vi "函数类型1测试.vi"() -> ()   [LabVIEW 2010]
uses:
  全局量/试验配置信息.vi
panel:
  out "starttest":bool
  out "bRece":bool
  out "bSend":bool
  out "D_IN_1":string[][](table) caption="表格"
  in  "加载文件名称":string
  out "配置文件路径":path
  out "配置文件目录":path
  in  "同步_1":i32
  in  "数组_反馈值":dbl[][](array[numeric])
  in  "第几个数据":i32
  in  "第几组数据":i32
  in  "数组_设定值":dbl[][](array[numeric])
  in  "数组_选择":bool[](array[boolean])
  out "light_32":bool
  out "light_31":bool
  out "light_30":bool
  out "light_29":bool
  out "light_28":bool
  out "light_27":bool
  out "light_26":bool
  out "light_25":bool
  out "light_24":bool
  out "light_23":bool
  out "light_22":bool
  out "light_21":bool
  out "light_20":bool
  out "light_19":bool
  out "light_18":bool
  out "light_17":bool
  out "Analog_back":string[][](table) caption="表格"
  in  "A_32":bool
  in  "A_31":bool
  in  "A_30":bool
  in  "A_29":bool
  in  "A_28":bool
  in  "A_27":bool
  in  "A_26":bool
  in  "A_25":bool
  in  "A_24":bool
  in  "A_23":bool
  in  "A_22":bool
  in  "A_21":bool
  in  "A_20":bool
  in  "A_19":bool
  in  "A_18":bool
  in  "A_17":bool
  out "合格？":bool[][](array[boolean])
  out "测试结论":string
  out "light_16":bool
  out "light_15":bool
  out "light_14":bool
  out "light_13":bool
  out "light_12":bool
  out "light_11":bool
  out "light_10":bool
  out "light_9":bool
  out "light_8":bool
  out "light_7":bool
  out "light_6":bool
  out "light_5":bool
  out "light_4":bool
  out "light_3":bool
  out "light_2":bool
  out "light_1":bool
  out "退出？":bool
  in  "btn_反选":bool
  in  "btn_全选":bool
  in  "A_16":bool
  in  "A_15":bool
  in  "A_14":bool
  in  "A_13":bool
  in  "A_12":bool
  in  "A_11":bool
  in  "A_10":bool
  in  "A_9":bool
  in  "A_8":bool
  in  "A_7":bool
  in  "A_6":bool
  in  "A_5":bool
  in  "A_4":bool
  in  "A_3":bool
  in  "A_2":bool
  in  "A_1":bool
  in  "btn_取消":bool
  in  "btn_开始测试":bool
  in  "Analog_IN":string[][](table) caption="表格"
  out "Analog_WC":string[][](table) caption="表格"
  # "模拟量选择及输入值（V）"
  # "模拟量反馈值（V）"
  # "模拟量误差值（%）"
  # "测试结论："
  # "从0开始"
  # "从1开始,第0列没有使用"
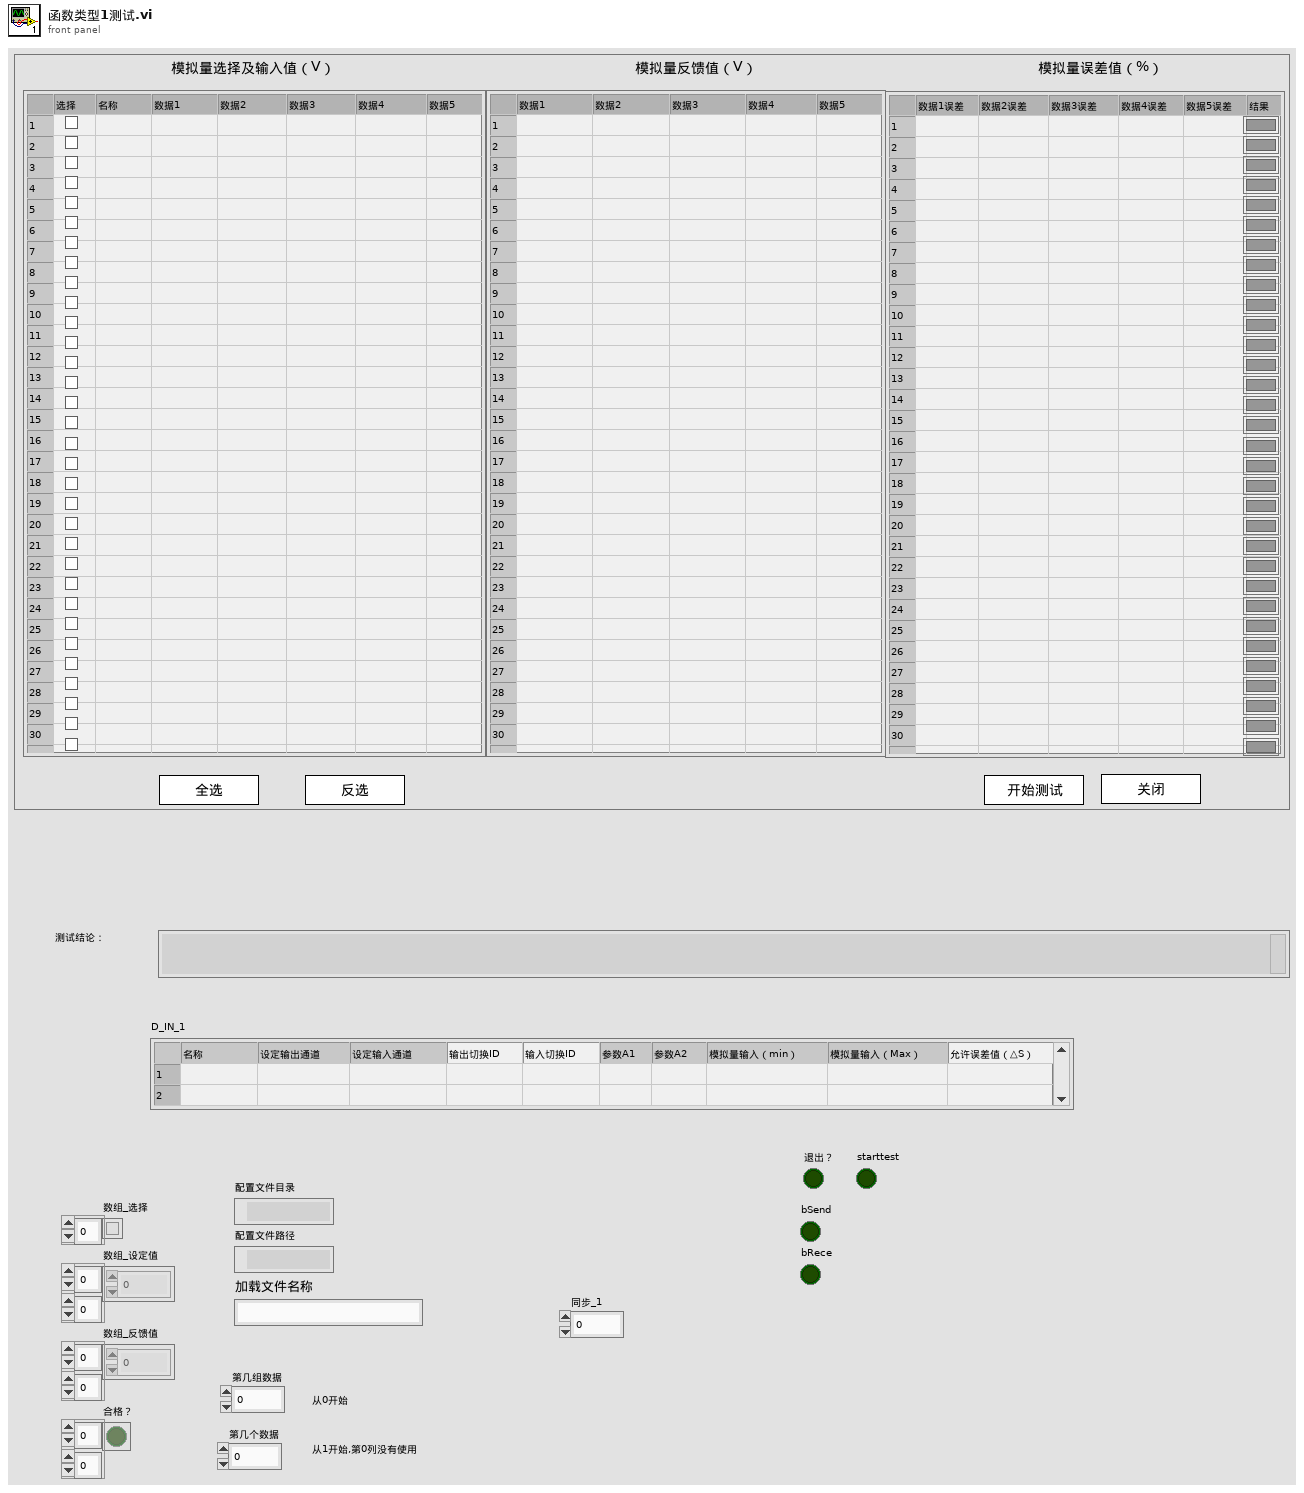
[diagram p1: front panel]
types:
  T1 = enum8{"Enabled", "Disabled", "Disabled and Grayed Out"}
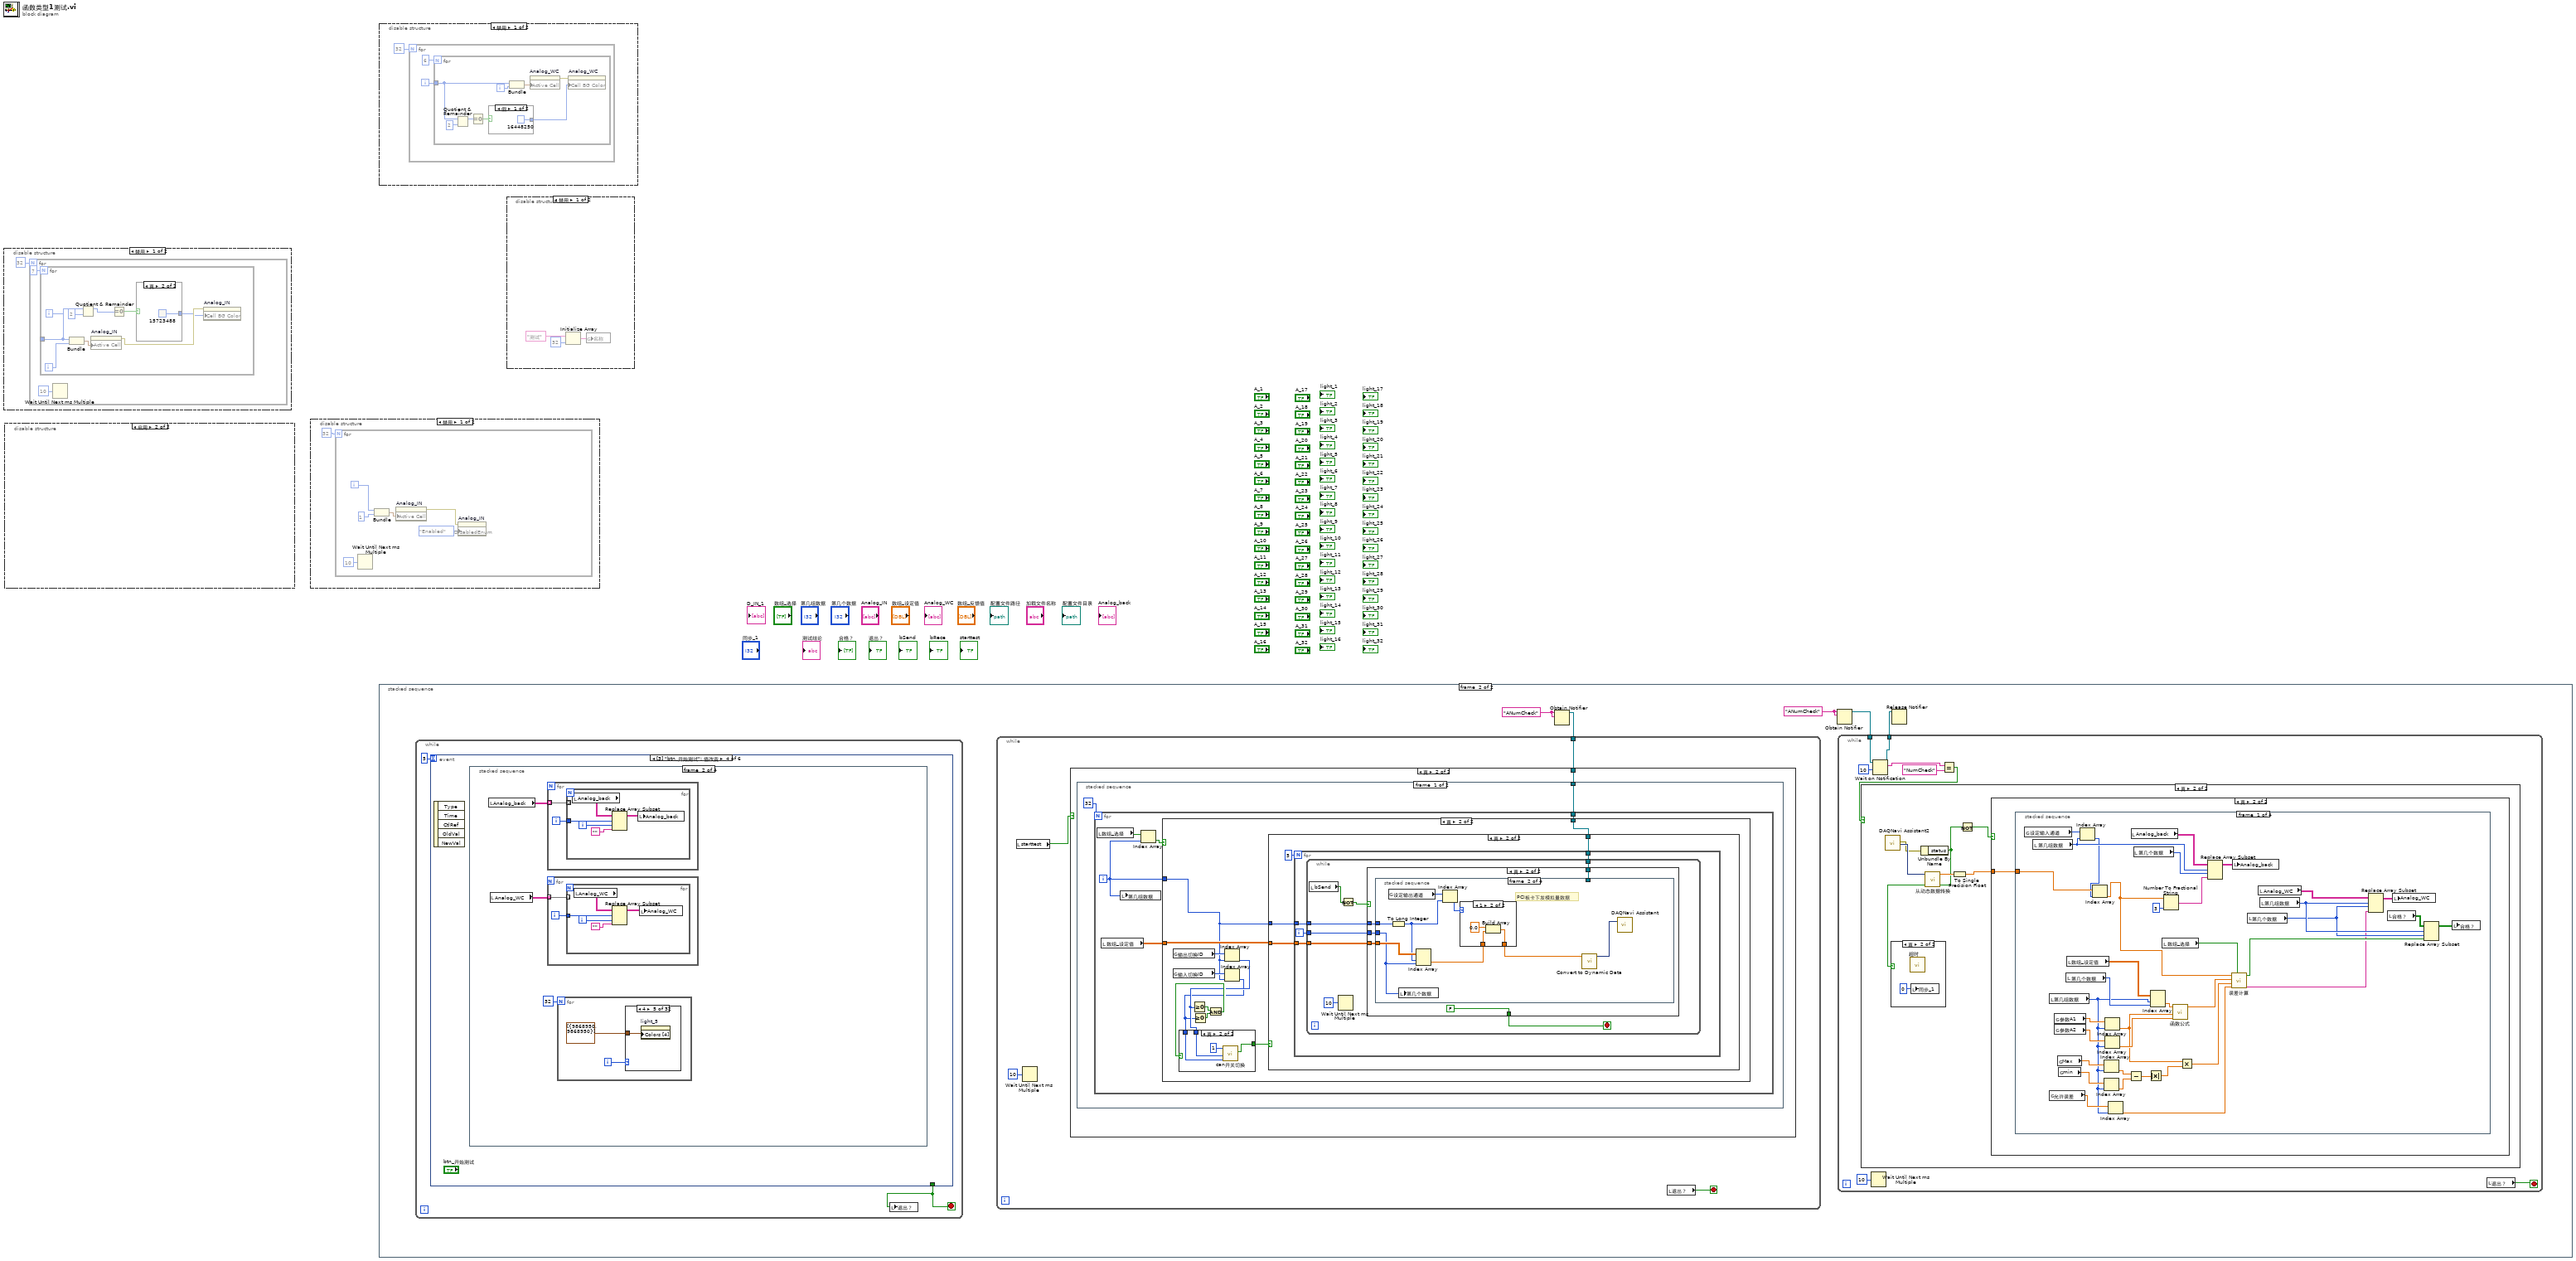
[diagram p0: block diagram]
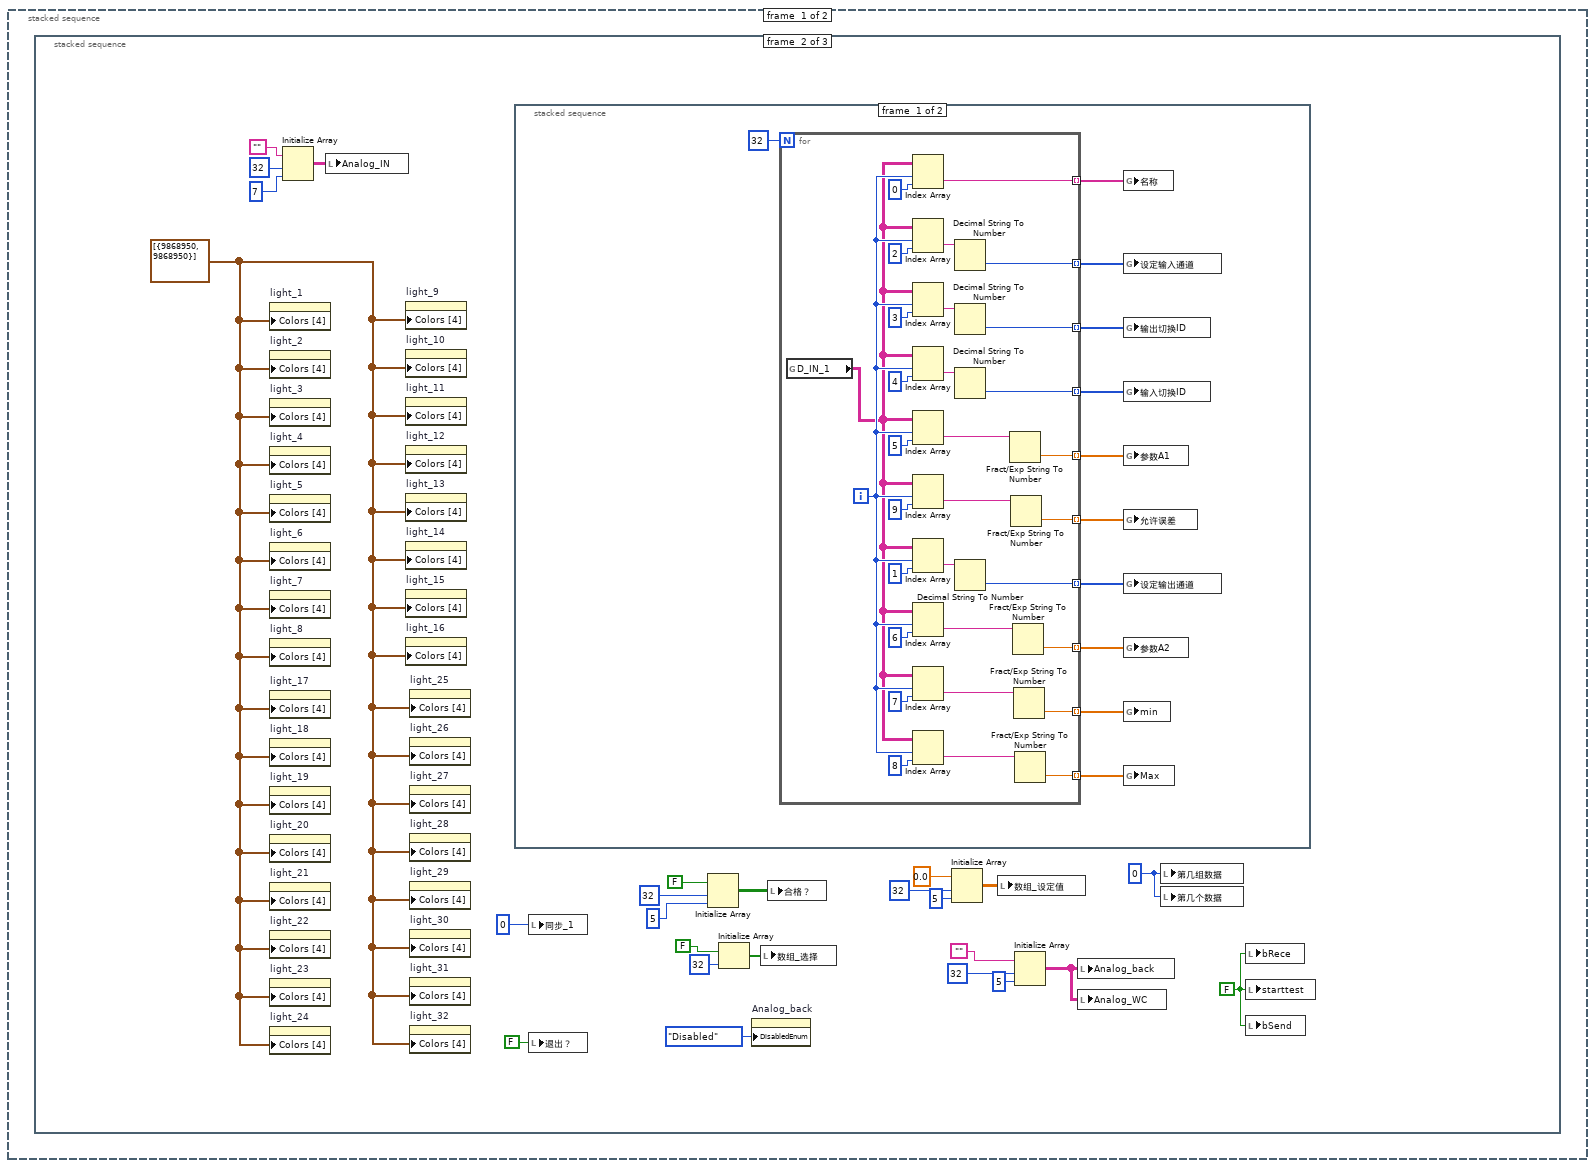
[diagram p2: hidden frame]
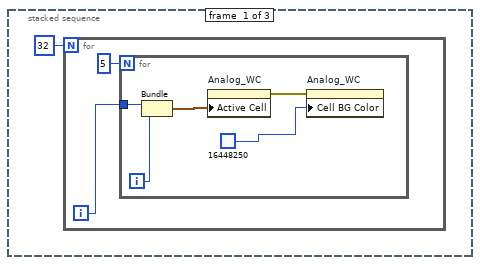
[diagram p3: hidden frame]
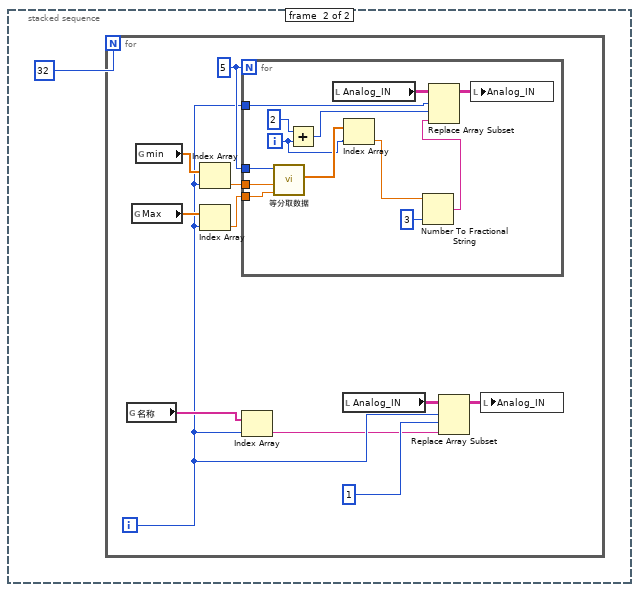
[diagram p4: hidden frame]
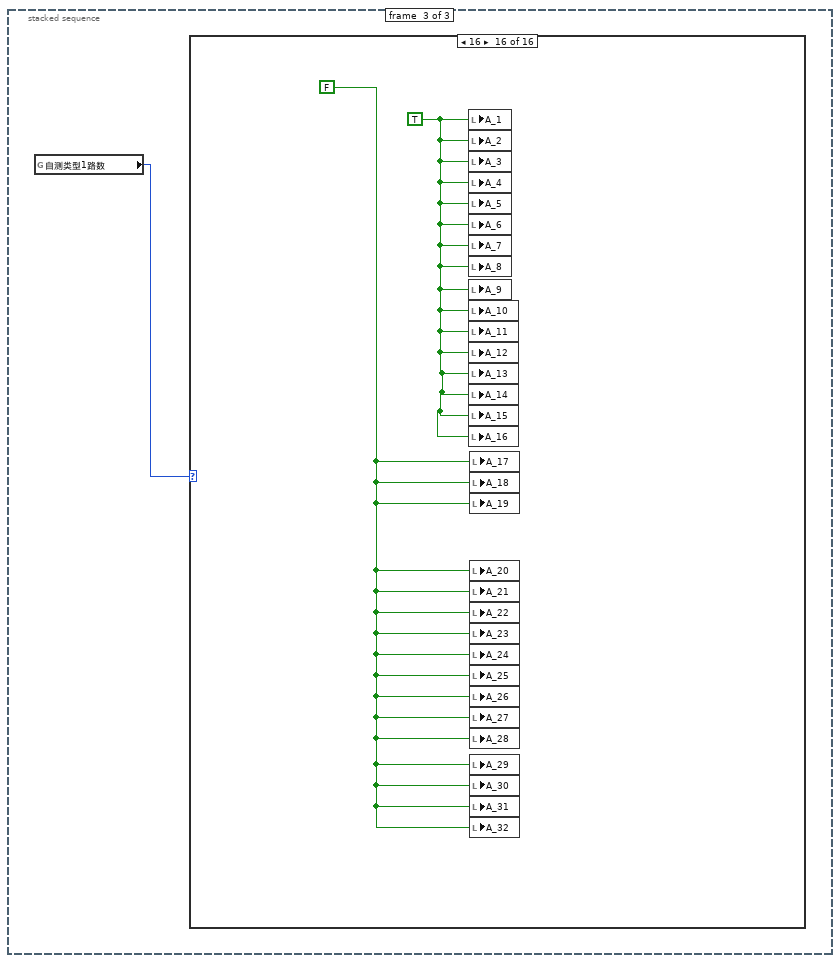
[diagram p5: hidden frame]
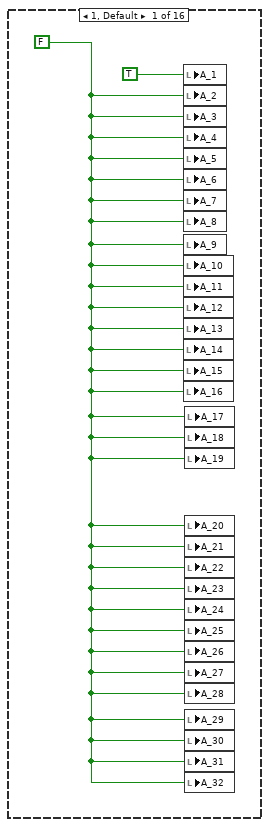
[diagram p6: hidden frame]
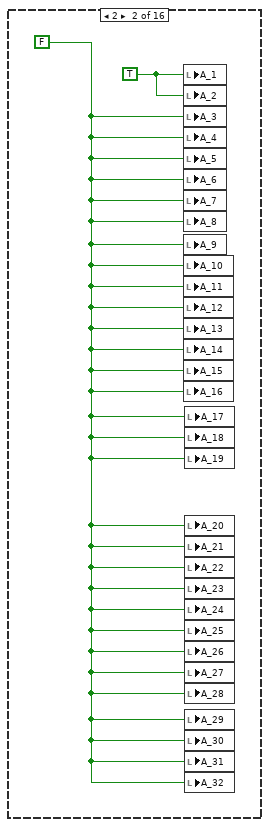
[diagram p7: hidden frame]
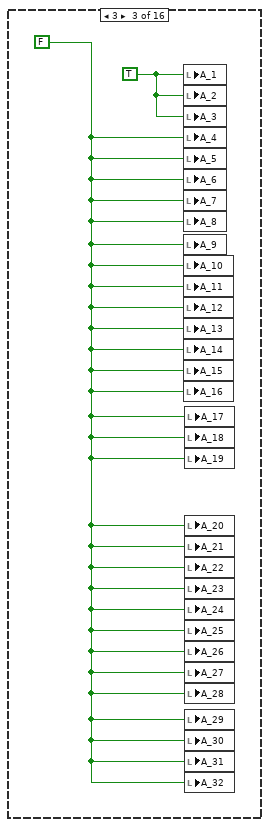
[diagram p8: hidden frame]
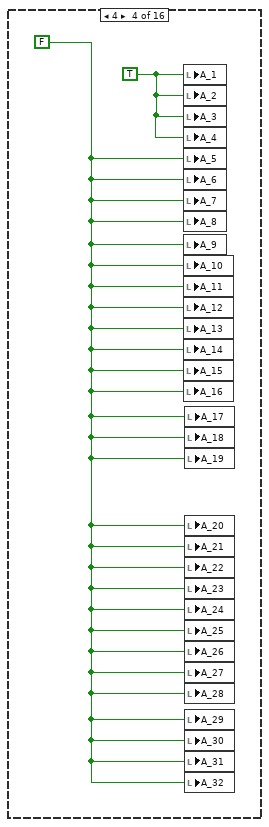
[diagram p9: hidden frame]
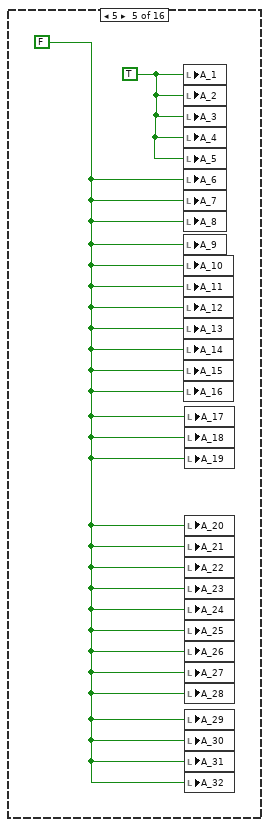
[diagram p10: hidden frame]
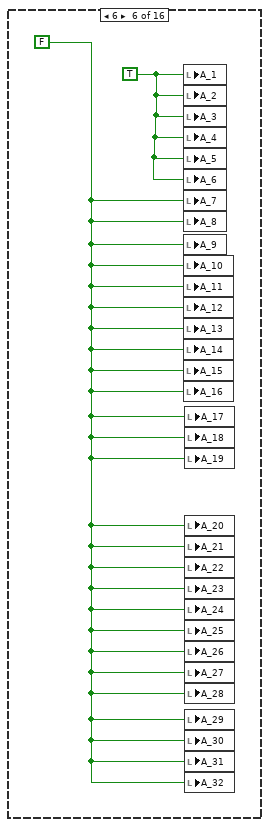
[diagram p11: hidden frame]
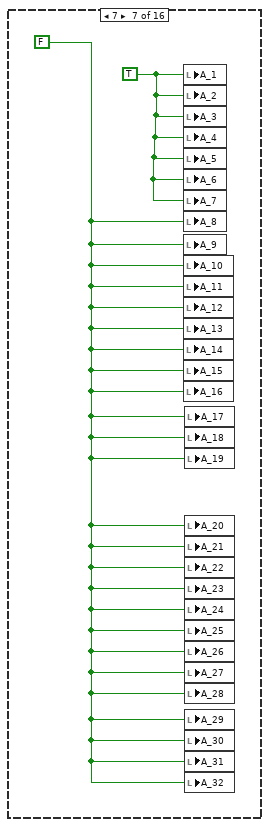
[diagram p12: hidden frame]
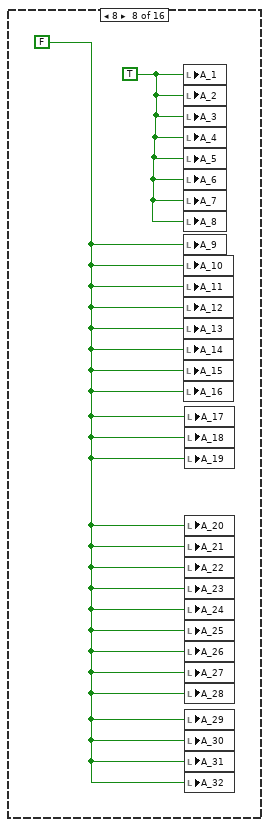
[diagram p13: hidden frame]
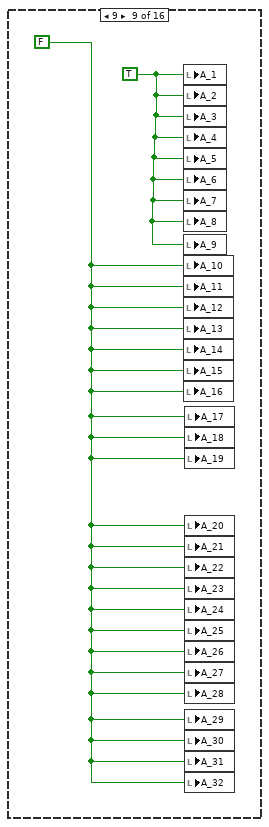
[diagram p14: hidden frame]
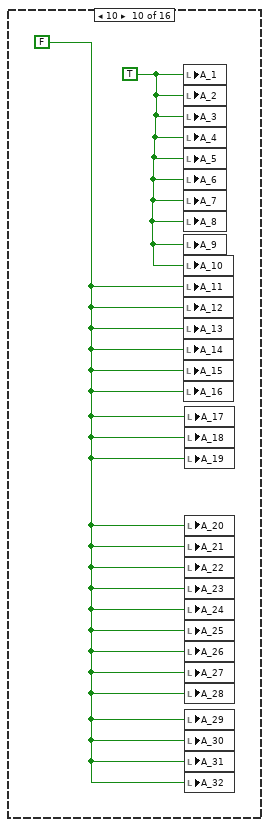
[diagram p15: hidden frame]
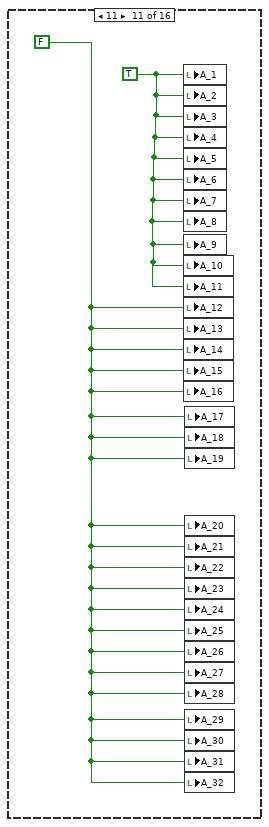
[diagram p16: hidden frame]
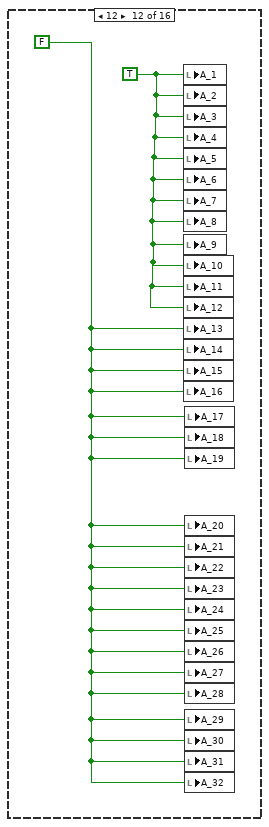
[diagram p17: hidden frame]
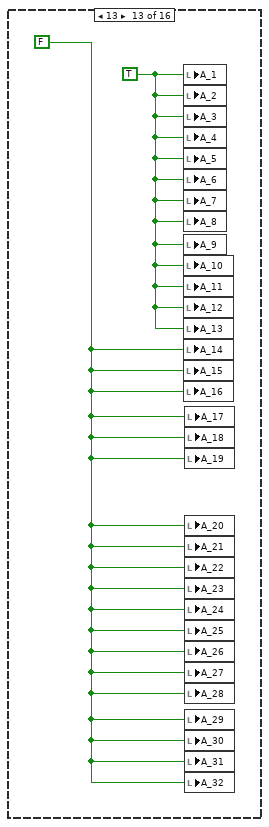
[diagram p18: hidden frame]
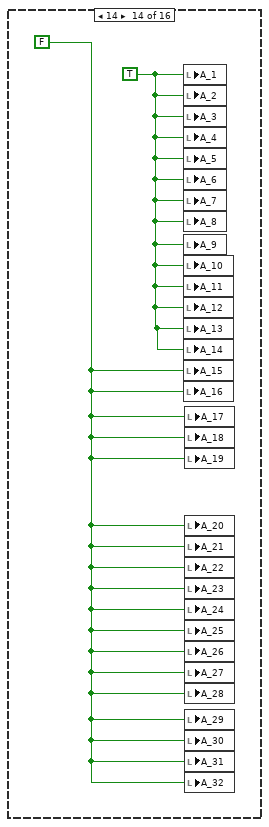
[diagram p19: hidden frame]
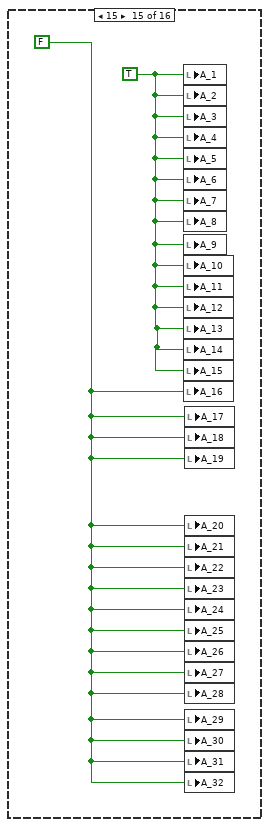
[diagram p20: hidden frame]
diagram:
  n1 = disable-structure shown="禁用" {
    frame Disabled {
      n2 = for {
        N: 32 -> [_]
        i -> [w3]
        n3 = for {
          N: 7 -> [_]
          tunnel: w3 -> [w11]
          i -> [w5]
          n4 = Bundle(w11, w5) -> (w8:cluster{i32, i32})  [unwired: 1 in]
          n5 = Quotient & Remainder(x=w11, y=2) -> (x-y*floor(x/y)=w9:i32)  [unwired: 1 out]
          n6 = property on="Analog_IN" class="Tbl (严格)"("Active Cell"=w8) -> (error out=w7:errorcluster)  [unwired: 2 in, 1 out]
          n7 = Equal To 0?(x=w9) -> (x = 0?=w12:bool)
          n8 = case shown="真" w12 {
            tunnel: [u32 16448250 u32 15723488] -> w6
            frame False {
            }
            frame True {
            }
          }
          n9 = property on="Analog_IN" class="Tbl (严格)"(error in=w7, "Cell BG Color"=w6) -> ()  [unwired: 1 in, 2 out]
        }
        n10 = Wait Until Next ms Multiple(millisecond multiple=u32 10 ("毫秒倍数")) -> ()  [unwired: 1 out]
      }
    }
    frame Enabled {
    }
  }
  n11 = disable-structure shown="启用" {
    frame Disabled {
      n12 = for {
        N: 32 -> [_]
        i -> [w16]
        n13 = for {
          N: 7 -> [_]
          tunnel: w16 -> [w19]
          i -> [w20]
          n14 = Bundle(w19, w20) -> (w23:cluster{i32, i32})  [unwired: 1 in]
          n15 = property on="Analog_IN" class="Tbl (严格)"("Active Cell"=w23) -> (error out=w21:errorcluster)  [unwired: 2 in, 1 out]
          n16 = property on="Analog_IN" class="Tbl (严格)"(error in=w21, "Justify"=enum16{"Left", "Center", "Right"}."Left" ("活动单元格:单元格对齐")) -> ()  [unwired: 1 in, 2 out]
        }
        n17 = Wait Until Next ms Multiple(millisecond multiple=u32 10 ("毫秒倍数")) -> ()  [unwired: 1 out]
      }
    }
    frame Enabled {
    }
  }
  n18 = disable-structure shown="禁用" {
    frame Disabled {
      n19 = for {
        N: 32 -> [_]
        i -> [w29]
        n20 = Wait Until Next ms Multiple(millisecond multiple=u32 10 ("毫秒倍数")) -> ()  [unwired: 1 out]
        n21 = Bundle(w29, 1) -> (w28:cluster{i32, i32})  [unwired: 1 in]
        n22 = property on="Analog_IN" class="Tbl (严格)"("Active Cell"=w28) -> (error out=w25:errorcluster)  [unwired: 2 in, 1 out]
        n23 = property on="Analog_IN" class="Tbl (严格)"(error in=w25, "DisabledEnum"=T1."Enabled" ("禁用")) -> ()  [unwired: 1 in, 2 out]
      }
    }
    frame Enabled {
    }
  }
  n24 = stacked-sequence {
    frame #0 {
      n25 = stacked-sequence {
        frame #0 {
          n26 = for {
            N: 32 -> [_]
            i -> [w32]
            n27 = for {
              N: 5 -> [_]
              tunnel: w32 -> [w35]
              i -> [w34]
              n28 = Bundle(w35, w34) -> (w36:cluster{i32, i32})  [unwired: 1 in]
              n29 = property on="Analog_WC" class="Tbl (严格)"("Active Cell"=w36) -> (error out=w38:errorcluster)  [unwired: 2 in, 1 out]
              n30 = property on="Analog_WC" class="Tbl (严格)"(error in=w38, "Cell BG Color"=u32 16448250) -> ()  [unwired: 1 in, 2 out]
            }
          }
        }
        frame #1 {
          w63 = FALSE
          w58 = 0 ("第几组数据")
          w43 = cluster{u32, u32}[] [{9868950, 9868950}]
          n31 = property on="light_1" class="Bool (严格)"("Colors [4]"=w43) -> ()  [unwired: 2 in, 2 out]
          n32 = property on="light_2" class="Bool (严格)"("Colors [4]"=w43) -> ()  [unwired: 2 in, 2 out]
          n33 = property on="light_3" class="Bool (严格)"("Colors [4]"=w43) -> ()  [unwired: 2 in, 2 out]
          n34 = property on="light_4" class="Bool (严格)"("Colors [4]"=w43) -> ()  [unwired: 2 in, 2 out]
          n35 = property on="light_5" class="Bool (严格)"("Colors [4]"=w43) -> ()  [unwired: 2 in, 2 out]
          n36 = property on="light_6" class="Bool (严格)"("Colors [4]"=w43) -> ()  [unwired: 2 in, 2 out]
          n37 = property on="light_7" class="Bool (严格)"("Colors [4]"=w43) -> ()  [unwired: 2 in, 2 out]
          n38 = property on="light_8" class="Bool (严格)"("Colors [4]"=w43) -> ()  [unwired: 2 in, 2 out]
          n39 = property on="light_17" class="Bool (严格)"("Colors [4]"=w43) -> ()  [unwired: 2 in, 2 out]
          n40 = property on="light_18" class="Bool (严格)"("Colors [4]"=w43) -> ()  [unwired: 2 in, 2 out]
          n41 = property on="light_19" class="Bool (严格)"("Colors [4]"=w43) -> ()  [unwired: 2 in, 2 out]
          n42 = property on="light_20" class="Bool (严格)"("Colors [4]"=w43) -> ()  [unwired: 2 in, 2 out]
          n43 = property on="light_21" class="Bool (严格)"("Colors [4]"=w43) -> ()  [unwired: 2 in, 2 out]
          n44 = property on="light_22" class="Bool (严格)"("Colors [4]"=w43) -> ()  [unwired: 2 in, 2 out]
          n45 = property on="light_23" class="Bool (严格)"("Colors [4]"=w43) -> ()  [unwired: 2 in, 2 out]
          n46 = property on="light_24" class="Bool (严格)"("Colors [4]"=w43) -> ()  [unwired: 2 in, 2 out]
          n47 = Initialize Array("", 32 ("维数大小"), 7 ("维数大小")) -> (w59:string[][])
          n48 = local write "Analog_IN"(w59) -> ()
          n49 = property on="light_9" class="Bool (严格)"("Colors [4]"=w43) -> ()  [unwired: 2 in, 2 out]
          n50 = property on="light_10" class="Bool (严格)"("Colors [4]"=w43) -> ()  [unwired: 2 in, 2 out]
          n51 = property on="light_11" class="Bool (严格)"("Colors [4]"=w43) -> ()  [unwired: 2 in, 2 out]
          n52 = property on="light_12" class="Bool (严格)"("Colors [4]"=w43) -> ()  [unwired: 2 in, 2 out]
          n53 = property on="light_13" class="Bool (严格)"("Colors [4]"=w43) -> ()  [unwired: 2 in, 2 out]
          n54 = property on="light_14" class="Bool (严格)"("Colors [4]"=w43) -> ()  [unwired: 2 in, 2 out]
          n55 = property on="light_15" class="Bool (严格)"("Colors [4]"=w43) -> ()  [unwired: 2 in, 2 out]
          n56 = property on="light_16" class="Bool (严格)"("Colors [4]"=w43) -> ()  [unwired: 2 in, 2 out]
          n57 = property on="light_25" class="Bool (严格)"("Colors [4]"=w43) -> ()  [unwired: 2 in, 2 out]
          n58 = property on="light_26" class="Bool (严格)"("Colors [4]"=w43) -> ()  [unwired: 2 in, 2 out]
          n59 = property on="light_27" class="Bool (严格)"("Colors [4]"=w43) -> ()  [unwired: 2 in, 2 out]
          n60 = property on="light_28" class="Bool (严格)"("Colors [4]"=w43) -> ()  [unwired: 2 in, 2 out]
          n61 = property on="light_29" class="Bool (严格)"("Colors [4]"=w43) -> ()  [unwired: 2 in, 2 out]
          n62 = property on="light_30" class="Bool (严格)"("Colors [4]"=w43) -> ()  [unwired: 2 in, 2 out]
          n63 = property on="light_31" class="Bool (严格)"("Colors [4]"=w43) -> ()  [unwired: 2 in, 2 out]
          n64 = property on="light_32" class="Bool (严格)"("Colors [4]"=w43) -> ()  [unwired: 2 in, 2 out]
          n65 = stacked-sequence {
            frame #0 {
              n66 = for {
                N: 32 ("维数大小") -> [_]
                tunnel: [w104] -> w68 mode=indexing
                tunnel: [w100] -> w67 mode=indexing
                tunnel: [w98] -> w66 mode=indexing
                tunnel: [w95] -> w65 mode=indexing
                tunnel: [w92] -> w64 mode=indexing
                tunnel: [w89] -> w70 mode=indexing
                tunnel: [w86] -> w71 mode=indexing
                tunnel: [w83] -> w72 mode=indexing
                tunnel: [w80] -> w73 mode=indexing
                tunnel: [w76] -> w74 mode=indexing
                i -> [w78]
                n67 = global read "试验配置信息.vi" "D_IN_1"() -> (w75:string[][])
                n68 = Index Array(array=w75, index (row)=w78, index (col)=0 ("禁用的索引 (列)")) -> (element=w104:string)
                n69 = Index Array(array=w75, index (row)=w78, index (col)=2 ("禁用的索引 (列)")) -> (element=w94:string)
                n70 = Index Array(array=w75, index (row)=w78, index (col)=3 ("禁用的索引 (列)")) -> (element=w90:string)
                n71 = Index Array(array=w75, index (row)=w78, index (col)=4 ("禁用的索引 (列)")) -> (element=w88:string)
                n72 = Index Array(array=w75, index (row)=w78, index (col)=5 ("禁用的索引 (列)")) -> (element=w85:string)
                n73 = Index Array(array=w75, index (row)=w78, index (col)=9 ("禁用的索引 (列)")) -> (element=w77:string)
                n74 = Index Array(array=w75, index (row)=w78, index (col)=1 ("禁用的索引 (列)")) -> (element=w97:string)
                n75 = Index Array(array=w75, index (row)=w78, index (col)=6 ("禁用的索引 (列)")) -> (element=w81:string)
                n76 = Index Array(array=w75, index (row)=w78, index (col)=7 ("禁用的索引 (列)")) -> (element=w101:string)
                n77 = Index Array(array=w75, index (row)=w78, index (col)=8 ("禁用的索引 (列)")) -> (element=w99:string)
                n78 = Decimal String To Number(string=w94) -> (number=w92:i32)  [unwired: 2 in, 1 out]
                n79 = Decimal String To Number(string=w90) -> (number=w89:i32)  [unwired: 2 in, 1 out]
                n80 = Decimal String To Number(string=w88) -> (number=w86:i32)  [unwired: 2 in, 1 out]
                n81 = Decimal String To Number(string=w97) -> (number=w95:i32)  [unwired: 2 in, 1 out]
                n82 = Fract/Exp String To Number(string=w85) -> (number=w83:dbl)  [unwired: 3 in, 1 out]
                n83 = Fract/Exp String To Number(string=w77) -> (number=w76:dbl)  [unwired: 3 in, 1 out]
                n84 = Fract/Exp String To Number(string=w81) -> (number=w80:dbl)  [unwired: 3 in, 1 out]
                n85 = Fract/Exp String To Number(string=w101) -> (number=w100:dbl)  [unwired: 3 in, 1 out]
                n86 = Fract/Exp String To Number(string=w99) -> (number=w98:dbl)  [unwired: 3 in, 1 out]
              }
              n87 = global write "试验配置信息.vi" "名称"(w68) -> ()
              n88 = global write "试验配置信息.vi" "设定输入通道"(w64) -> ()
              n89 = global write "试验配置信息.vi" "输出切换ID"(w70) -> ()
              n90 = global write "试验配置信息.vi" "输入切换ID"(w71) -> ()
              n91 = global write "试验配置信息.vi" "参数A1"(w72) -> ()
              n92 = global write "试验配置信息.vi" "允许误差"(w74) -> ()
              n93 = global write "试验配置信息.vi" "设定输出通道"(w65) -> ()
              n94 = global write "试验配置信息.vi" "参数A2"(w73) -> ()
              n95 = global write "试验配置信息.vi" "min"(w67) -> ()
              n96 = global write "试验配置信息.vi" "Max"(w66) -> ()
            }
            frame #1 {
              n97 = for {
                N: 32 -> [_]
                i -> [w109]
                w113 = 5 ("num")
                n98 = global read "试验配置信息.vi" "名称"() -> (w112:string[])
                n99 = global read "试验配置信息.vi" "Max"() -> (w116:dbl[])
                n100 = global read "试验配置信息.vi" "min"() -> (w117:dbl[])
                n101 = Index Array(array=w117, index=w109) -> (element=w115:dbl)
                n102 = Index Array(array=w116, index=w109) -> (element=w114:dbl)
                n103 = for {
                  N: w113 -> [_]
                  tunnel: w109 -> [w128]
                  tunnel: w115 -> [w125]
                  tunnel: w114 -> [w124]
                  tunnel: w113 -> [w123]
                  i -> [w121]
                  n104 = call "等分取数据.vi"("Max"=w124, "MIN"=w125, "num"=w123) -> ("数据点"=w122:dbl[])  [unwired: 5 in]
                  n105 = Add(x=2, y=w121) -> (x+y=w126:i32)
                  n106 = local read "Analog_IN"() -> (w130:string[][])
                  n107 = Index Array(array=w122, index=w121) -> (element=w119:dbl)
                  n108 = Number To Fractional String(number=w119, precision (6)=i16 3 ("精度(6)")) -> (F-format string=w120:string)  [unwired: 2 in]
                  n109 = Replace Array Subset(array=w130, new element=w120, index (row)=w128, index (col)=w126) -> (w129:string[][])
                  n110 = local write "Analog_IN"(w129) -> ()
                }
                n111 = Index Array(array=w112, index=w109) -> (element=w107:string)
                n112 = local read "Analog_IN"() -> (w110:string[][])
                n113 = Replace Array Subset(array=w110, new element=w107, index (row)=w109, index (col)=1) -> (w111:string[][])
                n114 = local write "Analog_IN"(w111) -> ()
              }
            }
          }
          n115 = local write "同步_1"(0 ("同步_2")) -> ()
          n116 = local write "退出？"(FALSE ("退出？")) -> ()
          n117 = Initialize Array(FALSE, 32 ("维数大小"), 5 ("维数大小")) -> (w42:bool[][])
          n118 = Initialize Array(FALSE, 32 ("维数大小")) -> (w54:bool[])
          n119 = property on="Analog_back" class="Tbl (严格)"("DisabledEnum"=T1."Disabled" ("禁用")) -> ()  [unwired: 2 in, 2 out]
          n120 = local write "数组_选择"(w54) -> ()
          n121 = local write "合格？"(w42) -> ()
          n122 = Initialize Array(0.0, 32 ("维数大小"), 5 ("维数大小")) -> (w51:dbl[][])
          n123 = local write "数组_设定值"(w51) -> ()
          n124 = Initialize Array("", 32 ("维数大小"), 5 ("维数大小")) -> (w47:string[][])
          n125 = local write "Analog_back"(w47) -> ()
          n126 = local write "Analog_WC"(w47) -> ()
          n127 = local write "第几组数据"(w58) -> ()
          n128 = local write "第几个数据"(w58) -> ()
          n129 = local write "bRece"(w63) -> ()
          n130 = local write "starttest"(w63) -> ()
          n131 = local write "bSend"(w63) -> ()
        }
        frame #2 {
          n132 = global read "试验配置信息.vi" "自测类型1路数"() -> (w131:i32)
          n133 = case shown="16" w131 {
            frame 1, Default {
              w133 = FALSE ("单选_AD_1")
              n134 = local write "A_1"(TRUE) -> ()
              n135 = local write "A_2"(w133) -> ()
              n136 = local write "A_3"(w133) -> ()
              n137 = local write "A_4"(w133) -> ()
              n138 = local write "A_5"(w133) -> ()
              n139 = local write "A_6"(w133) -> ()
              n140 = local write "A_7"(w133) -> ()
              n141 = local write "A_8"(w133) -> ()
              n142 = local write "A_9"(w133) -> ()
              n143 = local write "A_10"(w133) -> ()
              n144 = local write "A_11"(w133) -> ()
              n145 = local write "A_12"(w133) -> ()
              n146 = local write "A_13"(w133) -> ()
              n147 = local write "A_14"(w133) -> ()
              n148 = local write "A_15"(w133) -> ()
              n149 = local write "A_16"(w133) -> ()
              n150 = local write "A_17"(w133) -> ()
              n151 = local write "A_18"(w133) -> ()
              n152 = local write "A_19"(w133) -> ()
              n153 = local write "A_20"(w133) -> ()
              n154 = local write "A_21"(w133) -> ()
              n155 = local write "A_22"(w133) -> ()
              n156 = local write "A_23"(w133) -> ()
              n157 = local write "A_24"(w133) -> ()
              n158 = local write "A_25"(w133) -> ()
              n159 = local write "A_26"(w133) -> ()
              n160 = local write "A_27"(w133) -> ()
              n161 = local write "A_28"(w133) -> ()
              n162 = local write "A_29"(w133) -> ()
              n163 = local write "A_30"(w133) -> ()
              n164 = local write "A_31"(w133) -> ()
              n165 = local write "A_32"(w133) -> ()
            }
            frame 2 {
              w134 = TRUE
              w135 = FALSE ("单选_AD_1")
              n166 = local write "A_1"(w134) -> ()
              n167 = local write "A_2"(w134) -> ()
              n168 = local write "A_3"(w135) -> ()
              n169 = local write "A_4"(w135) -> ()
              n170 = local write "A_5"(w135) -> ()
              n171 = local write "A_6"(w135) -> ()
              n172 = local write "A_7"(w135) -> ()
              n173 = local write "A_8"(w135) -> ()
              n174 = local write "A_9"(w135) -> ()
              n175 = local write "A_10"(w135) -> ()
              n176 = local write "A_11"(w135) -> ()
              n177 = local write "A_12"(w135) -> ()
              n178 = local write "A_13"(w135) -> ()
              n179 = local write "A_14"(w135) -> ()
              n180 = local write "A_15"(w135) -> ()
              n181 = local write "A_16"(w135) -> ()
              n182 = local write "A_17"(w135) -> ()
              n183 = local write "A_18"(w135) -> ()
              n184 = local write "A_19"(w135) -> ()
              n185 = local write "A_20"(w135) -> ()
              n186 = local write "A_21"(w135) -> ()
              n187 = local write "A_22"(w135) -> ()
              n188 = local write "A_23"(w135) -> ()
              n189 = local write "A_24"(w135) -> ()
              n190 = local write "A_25"(w135) -> ()
              n191 = local write "A_26"(w135) -> ()
              n192 = local write "A_27"(w135) -> ()
              n193 = local write "A_28"(w135) -> ()
              n194 = local write "A_29"(w135) -> ()
              n195 = local write "A_30"(w135) -> ()
              n196 = local write "A_31"(w135) -> ()
              n197 = local write "A_32"(w135) -> ()
            }
            frame 3 {
              w136 = TRUE
              w137 = FALSE ("单选_AD_1")
              n198 = local write "A_1"(w136) -> ()
              n199 = local write "A_2"(w136) -> ()
              n200 = local write "A_3"(w136) -> ()
              n201 = local write "A_4"(w137) -> ()
              n202 = local write "A_5"(w137) -> ()
              n203 = local write "A_6"(w137) -> ()
              n204 = local write "A_7"(w137) -> ()
              n205 = local write "A_8"(w137) -> ()
              n206 = local write "A_9"(w137) -> ()
              n207 = local write "A_10"(w137) -> ()
              n208 = local write "A_11"(w137) -> ()
              n209 = local write "A_12"(w137) -> ()
              n210 = local write "A_13"(w137) -> ()
              n211 = local write "A_14"(w137) -> ()
              n212 = local write "A_15"(w137) -> ()
              n213 = local write "A_16"(w137) -> ()
              n214 = local write "A_17"(w137) -> ()
              n215 = local write "A_18"(w137) -> ()
              n216 = local write "A_19"(w137) -> ()
              n217 = local write "A_20"(w137) -> ()
              n218 = local write "A_21"(w137) -> ()
              n219 = local write "A_22"(w137) -> ()
              n220 = local write "A_23"(w137) -> ()
              n221 = local write "A_24"(w137) -> ()
              n222 = local write "A_25"(w137) -> ()
              n223 = local write "A_26"(w137) -> ()
              n224 = local write "A_27"(w137) -> ()
              n225 = local write "A_28"(w137) -> ()
              n226 = local write "A_29"(w137) -> ()
              n227 = local write "A_30"(w137) -> ()
              n228 = local write "A_31"(w137) -> ()
              n229 = local write "A_32"(w137) -> ()
            }
            frame 4 {
              w138 = TRUE
              w139 = FALSE ("单选_AD_1")
              n230 = local write "A_1"(w138) -> ()
              n231 = local write "A_2"(w138) -> ()
              n232 = local write "A_3"(w138) -> ()
              n233 = local write "A_4"(w138) -> ()
              n234 = local write "A_5"(w139) -> ()
              n235 = local write "A_6"(w139) -> ()
              n236 = local write "A_7"(w139) -> ()
              n237 = local write "A_8"(w139) -> ()
              n238 = local write "A_9"(w139) -> ()
              n239 = local write "A_10"(w139) -> ()
              n240 = local write "A_11"(w139) -> ()
              n241 = local write "A_12"(w139) -> ()
              n242 = local write "A_13"(w139) -> ()
              n243 = local write "A_14"(w139) -> ()
              n244 = local write "A_15"(w139) -> ()
              n245 = local write "A_16"(w139) -> ()
              n246 = local write "A_17"(w139) -> ()
              n247 = local write "A_18"(w139) -> ()
              n248 = local write "A_19"(w139) -> ()
              n249 = local write "A_20"(w139) -> ()
              n250 = local write "A_21"(w139) -> ()
              n251 = local write "A_22"(w139) -> ()
              n252 = local write "A_23"(w139) -> ()
              n253 = local write "A_24"(w139) -> ()
              n254 = local write "A_25"(w139) -> ()
              n255 = local write "A_26"(w139) -> ()
              n256 = local write "A_27"(w139) -> ()
              n257 = local write "A_28"(w139) -> ()
              n258 = local write "A_29"(w139) -> ()
              n259 = local write "A_30"(w139) -> ()
              n260 = local write "A_31"(w139) -> ()
              n261 = local write "A_32"(w139) -> ()
            }
            frame 5 {
              w140 = TRUE
              w141 = FALSE ("单选_AD_1")
              n262 = local write "A_1"(w140) -> ()
              n263 = local write "A_2"(w140) -> ()
              n264 = local write "A_3"(w140) -> ()
              n265 = local write "A_4"(w140) -> ()
              n266 = local write "A_5"(w140) -> ()
              n267 = local write "A_6"(w141) -> ()
              n268 = local write "A_7"(w141) -> ()
              n269 = local write "A_8"(w141) -> ()
              n270 = local write "A_9"(w141) -> ()
              n271 = local write "A_10"(w141) -> ()
              n272 = local write "A_11"(w141) -> ()
              n273 = local write "A_12"(w141) -> ()
              n274 = local write "A_13"(w141) -> ()
              n275 = local write "A_14"(w141) -> ()
              n276 = local write "A_15"(w141) -> ()
              n277 = local write "A_16"(w141) -> ()
              n278 = local write "A_17"(w141) -> ()
              n279 = local write "A_18"(w141) -> ()
              n280 = local write "A_19"(w141) -> ()
              n281 = local write "A_20"(w141) -> ()
              n282 = local write "A_21"(w141) -> ()
              n283 = local write "A_22"(w141) -> ()
              n284 = local write "A_23"(w141) -> ()
              n285 = local write "A_24"(w141) -> ()
              n286 = local write "A_25"(w141) -> ()
              n287 = local write "A_26"(w141) -> ()
              n288 = local write "A_27"(w141) -> ()
              n289 = local write "A_28"(w141) -> ()
              n290 = local write "A_29"(w141) -> ()
              n291 = local write "A_30"(w141) -> ()
              n292 = local write "A_31"(w141) -> ()
              n293 = local write "A_32"(w141) -> ()
            }
            frame 6 {
              w142 = TRUE
              w143 = FALSE ("单选_AD_1")
              n294 = local write "A_1"(w142) -> ()
              n295 = local write "A_2"(w142) -> ()
              n296 = local write "A_3"(w142) -> ()
              n297 = local write "A_4"(w142) -> ()
              n298 = local write "A_5"(w142) -> ()
              n299 = local write "A_6"(w142) -> ()
              n300 = local write "A_7"(w143) -> ()
              n301 = local write "A_8"(w143) -> ()
              n302 = local write "A_9"(w143) -> ()
              n303 = local write "A_10"(w143) -> ()
              n304 = local write "A_11"(w143) -> ()
              n305 = local write "A_12"(w143) -> ()
              n306 = local write "A_13"(w143) -> ()
              n307 = local write "A_14"(w143) -> ()
              n308 = local write "A_15"(w143) -> ()
              n309 = local write "A_16"(w143) -> ()
              n310 = local write "A_17"(w143) -> ()
              n311 = local write "A_18"(w143) -> ()
              n312 = local write "A_19"(w143) -> ()
              n313 = local write "A_20"(w143) -> ()
              n314 = local write "A_21"(w143) -> ()
              n315 = local write "A_22"(w143) -> ()
              n316 = local write "A_23"(w143) -> ()
              n317 = local write "A_24"(w143) -> ()
              n318 = local write "A_25"(w143) -> ()
              n319 = local write "A_26"(w143) -> ()
              n320 = local write "A_27"(w143) -> ()
              n321 = local write "A_28"(w143) -> ()
              n322 = local write "A_29"(w143) -> ()
              n323 = local write "A_30"(w143) -> ()
              n324 = local write "A_31"(w143) -> ()
              n325 = local write "A_32"(w143) -> ()
            }
            frame 7 {
              w144 = TRUE
              w145 = FALSE ("单选_AD_1")
              n326 = local write "A_1"(w144) -> ()
              n327 = local write "A_2"(w144) -> ()
              n328 = local write "A_3"(w144) -> ()
              n329 = local write "A_4"(w144) -> ()
              n330 = local write "A_5"(w144) -> ()
              n331 = local write "A_6"(w144) -> ()
              n332 = local write "A_7"(w144) -> ()
              n333 = local write "A_8"(w145) -> ()
              n334 = local write "A_9"(w145) -> ()
              n335 = local write "A_10"(w145) -> ()
              n336 = local write "A_11"(w145) -> ()
              n337 = local write "A_12"(w145) -> ()
              n338 = local write "A_13"(w145) -> ()
              n339 = local write "A_14"(w145) -> ()
              n340 = local write "A_15"(w145) -> ()
              n341 = local write "A_16"(w145) -> ()
              n342 = local write "A_17"(w145) -> ()
              n343 = local write "A_18"(w145) -> ()
              n344 = local write "A_19"(w145) -> ()
              n345 = local write "A_20"(w145) -> ()
              n346 = local write "A_21"(w145) -> ()
              n347 = local write "A_22"(w145) -> ()
              n348 = local write "A_23"(w145) -> ()
              n349 = local write "A_24"(w145) -> ()
              n350 = local write "A_25"(w145) -> ()
              n351 = local write "A_26"(w145) -> ()
              n352 = local write "A_27"(w145) -> ()
              n353 = local write "A_28"(w145) -> ()
              n354 = local write "A_29"(w145) -> ()
              n355 = local write "A_30"(w145) -> ()
              n356 = local write "A_31"(w145) -> ()
              n357 = local write "A_32"(w145) -> ()
            }
            frame 8 {
              w146 = TRUE
              w147 = FALSE ("单选_AD_1")
              n358 = local write "A_1"(w146) -> ()
              n359 = local write "A_2"(w146) -> ()
              n360 = local write "A_3"(w146) -> ()
              n361 = local write "A_4"(w146) -> ()
              n362 = local write "A_5"(w146) -> ()
              n363 = local write "A_6"(w146) -> ()
              n364 = local write "A_7"(w146) -> ()
              n365 = local write "A_8"(w146) -> ()
              n366 = local write "A_9"(w147) -> ()
              n367 = local write "A_10"(w147) -> ()
              n368 = local write "A_11"(w147) -> ()
              n369 = local write "A_12"(w147) -> ()
              n370 = local write "A_13"(w147) -> ()
              n371 = local write "A_14"(w147) -> ()
              n372 = local write "A_15"(w147) -> ()
              n373 = local write "A_16"(w147) -> ()
              n374 = local write "A_17"(w147) -> ()
              n375 = local write "A_18"(w147) -> ()
              n376 = local write "A_19"(w147) -> ()
              n377 = local write "A_20"(w147) -> ()
              n378 = local write "A_21"(w147) -> ()
              n379 = local write "A_22"(w147) -> ()
              n380 = local write "A_23"(w147) -> ()
              n381 = local write "A_24"(w147) -> ()
              n382 = local write "A_25"(w147) -> ()
              n383 = local write "A_26"(w147) -> ()
              n384 = local write "A_27"(w147) -> ()
              n385 = local write "A_28"(w147) -> ()
              n386 = local write "A_29"(w147) -> ()
              n387 = local write "A_30"(w147) -> ()
              n388 = local write "A_31"(w147) -> ()
              n389 = local write "A_32"(w147) -> ()
            }
            frame 9 {
              w148 = TRUE
              w149 = FALSE ("单选_AD_1")
              n390 = local write "A_1"(w148) -> ()
              n391 = local write "A_2"(w148) -> ()
              n392 = local write "A_3"(w148) -> ()
              n393 = local write "A_4"(w148) -> ()
              n394 = local write "A_5"(w148) -> ()
              n395 = local write "A_6"(w148) -> ()
              n396 = local write "A_7"(w148) -> ()
              n397 = local write "A_8"(w148) -> ()
              n398 = local write "A_9"(w148) -> ()
              n399 = local write "A_10"(w149) -> ()
              n400 = local write "A_11"(w149) -> ()
              n401 = local write "A_12"(w149) -> ()
              n402 = local write "A_13"(w149) -> ()
              n403 = local write "A_14"(w149) -> ()
              n404 = local write "A_15"(w149) -> ()
              n405 = local write "A_16"(w149) -> ()
              n406 = local write "A_17"(w149) -> ()
              n407 = local write "A_18"(w149) -> ()
              n408 = local write "A_19"(w149) -> ()
              n409 = local write "A_20"(w149) -> ()
              n410 = local write "A_21"(w149) -> ()
              n411 = local write "A_22"(w149) -> ()
              n412 = local write "A_23"(w149) -> ()
              n413 = local write "A_24"(w149) -> ()
              n414 = local write "A_25"(w149) -> ()
              n415 = local write "A_26"(w149) -> ()
              n416 = local write "A_27"(w149) -> ()
              n417 = local write "A_28"(w149) -> ()
              n418 = local write "A_29"(w149) -> ()
              n419 = local write "A_30"(w149) -> ()
              n420 = local write "A_31"(w149) -> ()
              n421 = local write "A_32"(w149) -> ()
            }
            frame 10 {
              w150 = TRUE
              w151 = FALSE ("单选_AD_1")
              n422 = local write "A_1"(w150) -> ()
              n423 = local write "A_2"(w150) -> ()
              n424 = local write "A_3"(w150) -> ()
              n425 = local write "A_4"(w150) -> ()
              n426 = local write "A_5"(w150) -> ()
              n427 = local write "A_6"(w150) -> ()
              n428 = local write "A_7"(w150) -> ()
              n429 = local write "A_8"(w150) -> ()
              n430 = local write "A_9"(w150) -> ()
              n431 = local write "A_10"(w150) -> ()
              n432 = local write "A_11"(w151) -> ()
              n433 = local write "A_12"(w151) -> ()
              n434 = local write "A_13"(w151) -> ()
              n435 = local write "A_14"(w151) -> ()
              n436 = local write "A_15"(w151) -> ()
              n437 = local write "A_16"(w151) -> ()
              n438 = local write "A_17"(w151) -> ()
              n439 = local write "A_18"(w151) -> ()
              n440 = local write "A_19"(w151) -> ()
              n441 = local write "A_20"(w151) -> ()
              n442 = local write "A_21"(w151) -> ()
              n443 = local write "A_22"(w151) -> ()
              n444 = local write "A_23"(w151) -> ()
              n445 = local write "A_24"(w151) -> ()
              n446 = local write "A_25"(w151) -> ()
              n447 = local write "A_26"(w151) -> ()
              n448 = local write "A_27"(w151) -> ()
              n449 = local write "A_28"(w151) -> ()
              n450 = local write "A_29"(w151) -> ()
              n451 = local write "A_30"(w151) -> ()
              n452 = local write "A_31"(w151) -> ()
              n453 = local write "A_32"(w151) -> ()
            }
            frame 11 {
              w152 = TRUE
              w153 = FALSE ("单选_AD_1")
              n454 = local write "A_1"(w152) -> ()
              n455 = local write "A_2"(w152) -> ()
              n456 = local write "A_3"(w152) -> ()
              n457 = local write "A_4"(w152) -> ()
              n458 = local write "A_5"(w152) -> ()
              n459 = local write "A_6"(w152) -> ()
              n460 = local write "A_7"(w152) -> ()
              n461 = local write "A_8"(w152) -> ()
              n462 = local write "A_9"(w152) -> ()
              n463 = local write "A_10"(w152) -> ()
              n464 = local write "A_11"(w152) -> ()
              n465 = local write "A_12"(w153) -> ()
              n466 = local write "A_13"(w153) -> ()
              n467 = local write "A_14"(w153) -> ()
              n468 = local write "A_15"(w153) -> ()
              n469 = local write "A_16"(w153) -> ()
              n470 = local write "A_17"(w153) -> ()
              n471 = local write "A_18"(w153) -> ()
              n472 = local write "A_19"(w153) -> ()
              n473 = local write "A_20"(w153) -> ()
              n474 = local write "A_21"(w153) -> ()
              n475 = local write "A_22"(w153) -> ()
              n476 = local write "A_23"(w153) -> ()
              n477 = local write "A_24"(w153) -> ()
              n478 = local write "A_25"(w153) -> ()
              n479 = local write "A_26"(w153) -> ()
              n480 = local write "A_27"(w153) -> ()
              n481 = local write "A_28"(w153) -> ()
              n482 = local write "A_29"(w153) -> ()
              n483 = local write "A_30"(w153) -> ()
              n484 = local write "A_31"(w153) -> ()
              n485 = local write "A_32"(w153) -> ()
            }
            frame 12 {
              w154 = TRUE
              w155 = FALSE ("单选_AD_1")
              n486 = local write "A_1"(w154) -> ()
              n487 = local write "A_2"(w154) -> ()
              n488 = local write "A_3"(w154) -> ()
              n489 = local write "A_4"(w154) -> ()
              n490 = local write "A_5"(w154) -> ()
              n491 = local write "A_6"(w154) -> ()
              n492 = local write "A_7"(w154) -> ()
              n493 = local write "A_8"(w154) -> ()
              n494 = local write "A_9"(w154) -> ()
              n495 = local write "A_10"(w154) -> ()
              n496 = local write "A_11"(w154) -> ()
              n497 = local write "A_12"(w154) -> ()
              n498 = local write "A_13"(w155) -> ()
              n499 = local write "A_14"(w155) -> ()
              n500 = local write "A_15"(w155) -> ()
              n501 = local write "A_16"(w155) -> ()
              n502 = local write "A_17"(w155) -> ()
              n503 = local write "A_18"(w155) -> ()
              n504 = local write "A_19"(w155) -> ()
              n505 = local write "A_20"(w155) -> ()
              n506 = local write "A_21"(w155) -> ()
              n507 = local write "A_22"(w155) -> ()
              n508 = local write "A_23"(w155) -> ()
              n509 = local write "A_24"(w155) -> ()
              n510 = local write "A_25"(w155) -> ()
              n511 = local write "A_26"(w155) -> ()
              n512 = local write "A_27"(w155) -> ()
              n513 = local write "A_28"(w155) -> ()
              n514 = local write "A_29"(w155) -> ()
              n515 = local write "A_30"(w155) -> ()
              n516 = local write "A_31"(w155) -> ()
              n517 = local write "A_32"(w155) -> ()
            }
            frame 13 {
              w156 = TRUE
              w157 = FALSE ("单选_AD_1")
              n518 = local write "A_1"(w156) -> ()
              n519 = local write "A_2"(w156) -> ()
              n520 = local write "A_3"(w156) -> ()
              n521 = local write "A_4"(w156) -> ()
              n522 = local write "A_5"(w156) -> ()
              n523 = local write "A_6"(w156) -> ()
              n524 = local write "A_7"(w156) -> ()
              n525 = local write "A_8"(w156) -> ()
              n526 = local write "A_9"(w156) -> ()
              n527 = local write "A_10"(w156) -> ()
              n528 = local write "A_11"(w156) -> ()
              n529 = local write "A_12"(w156) -> ()
              n530 = local write "A_13"(w156) -> ()
              n531 = local write "A_14"(w157) -> ()
              n532 = local write "A_15"(w157) -> ()
              n533 = local write "A_16"(w157) -> ()
              n534 = local write "A_17"(w157) -> ()
              n535 = local write "A_18"(w157) -> ()
              n536 = local write "A_19"(w157) -> ()
              n537 = local write "A_20"(w157) -> ()
              n538 = local write "A_21"(w157) -> ()
              n539 = local write "A_22"(w157) -> ()
              n540 = local write "A_23"(w157) -> ()
              n541 = local write "A_24"(w157) -> ()
              n542 = local write "A_25"(w157) -> ()
              n543 = local write "A_26"(w157) -> ()
              n544 = local write "A_27"(w157) -> ()
              n545 = local write "A_28"(w157) -> ()
              n546 = local write "A_29"(w157) -> ()
              n547 = local write "A_30"(w157) -> ()
              n548 = local write "A_31"(w157) -> ()
              n549 = local write "A_32"(w157) -> ()
            }
            frame 14 {
              w158 = TRUE
              w159 = FALSE ("单选_AD_1")
              n550 = local write "A_1"(w158) -> ()
              n551 = local write "A_2"(w158) -> ()
              n552 = local write "A_3"(w158) -> ()
              n553 = local write "A_4"(w158) -> ()
              n554 = local write "A_5"(w158) -> ()
              n555 = local write "A_6"(w158) -> ()
              n556 = local write "A_7"(w158) -> ()
              n557 = local write "A_8"(w158) -> ()
              n558 = local write "A_9"(w158) -> ()
              n559 = local write "A_10"(w158) -> ()
              n560 = local write "A_11"(w158) -> ()
              n561 = local write "A_12"(w158) -> ()
              n562 = local write "A_13"(w158) -> ()
              n563 = local write "A_14"(w158) -> ()
              n564 = local write "A_15"(w159) -> ()
              n565 = local write "A_16"(w159) -> ()
              n566 = local write "A_17"(w159) -> ()
              n567 = local write "A_18"(w159) -> ()
              n568 = local write "A_19"(w159) -> ()
              n569 = local write "A_20"(w159) -> ()
              n570 = local write "A_21"(w159) -> ()
              n571 = local write "A_22"(w159) -> ()
              n572 = local write "A_23"(w159) -> ()
              n573 = local write "A_24"(w159) -> ()
              n574 = local write "A_25"(w159) -> ()
              n575 = local write "A_26"(w159) -> ()
              n576 = local write "A_27"(w159) -> ()
              n577 = local write "A_28"(w159) -> ()
              n578 = local write "A_29"(w159) -> ()
              n579 = local write "A_30"(w159) -> ()
              n580 = local write "A_31"(w159) -> ()
              n581 = local write "A_32"(w159) -> ()
            }
            frame 15 {
              w160 = TRUE
              w161 = FALSE ("单选_AD_1")
              n582 = local write "A_1"(w160) -> ()
              n583 = local write "A_2"(w160) -> ()
              n584 = local write "A_3"(w160) -> ()
              n585 = local write "A_4"(w160) -> ()
              n586 = local write "A_5"(w160) -> ()
              n587 = local write "A_6"(w160) -> ()
              n588 = local write "A_7"(w160) -> ()
              n589 = local write "A_8"(w160) -> ()
              n590 = local write "A_9"(w160) -> ()
              n591 = local write "A_10"(w160) -> ()
              n592 = local write "A_11"(w160) -> ()
              n593 = local write "A_12"(w160) -> ()
              n594 = local write "A_13"(w160) -> ()
              n595 = local write "A_14"(w160) -> ()
              n596 = local write "A_15"(w160) -> ()
              n597 = local write "A_16"(w161) -> ()
              n598 = local write "A_17"(w161) -> ()
              n599 = local write "A_18"(w161) -> ()
              n600 = local write "A_19"(w161) -> ()
              n601 = local write "A_20"(w161) -> ()
              n602 = local write "A_21"(w161) -> ()
              n603 = local write "A_22"(w161) -> ()
              n604 = local write "A_23"(w161) -> ()
              n605 = local write "A_24"(w161) -> ()
              n606 = local write "A_25"(w161) -> ()
              n607 = local write "A_26"(w161) -> ()
              n608 = local write "A_27"(w161) -> ()
              n609 = local write "A_28"(w161) -> ()
              n610 = local write "A_29"(w161) -> ()
              n611 = local write "A_30"(w161) -> ()
              n612 = local write "A_31"(w161) -> ()
              n613 = local write "A_32"(w161) -> ()
            }
            frame 16 {
              w162 = TRUE
              w163 = FALSE ("单选_AD_1")
              n614 = local write "A_1"(w162) -> ()
              n615 = local write "A_2"(w162) -> ()
              n616 = local write "A_3"(w162) -> ()
              n617 = local write "A_4"(w162) -> ()
              n618 = local write "A_5"(w162) -> ()
              n619 = local write "A_6"(w162) -> ()
              n620 = local write "A_7"(w162) -> ()
              n621 = local write "A_8"(w162) -> ()
              n622 = local write "A_9"(w162) -> ()
              n623 = local write "A_10"(w162) -> ()
              n624 = local write "A_11"(w162) -> ()
              n625 = local write "A_12"(w162) -> ()
              n626 = local write "A_13"(w162) -> ()
              n627 = local write "A_14"(w162) -> ()
              n628 = local write "A_15"(w162) -> ()
              n629 = local write "A_16"(w162) -> ()
              n630 = local write "A_17"(w163) -> ()
              n631 = local write "A_18"(w163) -> ()
              n632 = local write "A_19"(w163) -> ()
              n633 = local write "A_20"(w163) -> ()
              n634 = local write "A_21"(w163) -> ()
              n635 = local write "A_22"(w163) -> ()
              n636 = local write "A_23"(w163) -> ()
              n637 = local write "A_24"(w163) -> ()
              n638 = local write "A_25"(w163) -> ()
              n639 = local write "A_26"(w163) -> ()
              n640 = local write "A_27"(w163) -> ()
              n641 = local write "A_28"(w163) -> ()
              n642 = local write "A_29"(w163) -> ()
              n643 = local write "A_30"(w163) -> ()
              n644 = local write "A_31"(w163) -> ()
              n645 = local write "A_32"(w163) -> ()
            }
          }
        }
      }
    }
    frame #1 {
      w165 = "ANumCheck" ("名称（未命名）")
      w168 = "ANumCheck" ("名称（未命名）")
      n646 = while {
        stop <- w361 stop-if-true
        n647 = event shown="[3] \"btn_开始测试\": 值改变" {
          selector: _ -> [_ _ _ _ _ _]
          dyn-events: _ -> [_ _ _ _ _ _]
          timeout: 5 -> [_ _ _ _ _ _]
          tunnel: [_ TRUE TRUE _ _ _] -> w361
          event Timeout {
            n648 = event-data() -> ()  [unwired: 1 in, 2 out]
            n649 = Wait Until Next ms Multiple(millisecond multiple=u32 2 ("毫秒倍数")) -> ()  [unwired: 1 out]
          }
          event Panel Close {
            n650 = event-data() -> ()  [unwired: 1 in, 3 out]
          }
          event "btn_取消": Value Change {
            n651 = event-data() -> ()  [unwired: 1 in, 5 out]
          }
          event "btn_开始测试": Value Change {
            n652 = event-data() -> ()  [unwired: 1 in, 5 out]
            n653 = stacked-sequence {
              frame #0 {
                w366 = FALSE
                w371 = 0 ("第几组数据")
                # "测试期间不准退出防止程序卡死"
                n654 = local read "Analog_IN"() -> (w377:string[][])
                n655 = Delete From Array(array=w377, length=1 ("长度"), index (col)=0 ("禁用的索引 (列)")) -> (array with subset deleted=w369:string[][])  [unwired: 1 in, 1 out]
                n656 = Delete From Array(array=w369, length=1 ("长度"), index (col)=0 ("禁用的索引 (列)")) -> (array with subset deleted=w367:string[][])  [unwired: 1 in, 1 out]
                n657 = for {
                  N: 32 -> [_]
                  tunnel: w367 -> [w387] mode=indexing
                  tunnel: [w386] -> w376 mode=indexing
                  n658 = for {
                    N: 5 -> [_]
                    tunnel: w387 -> [w389] mode=indexing
                    tunnel: [w388] -> w386 mode=indexing
                    n659 = Fract/Exp String To Number(string=w389) -> (number=w388:dbl)  [unwired: 3 in, 1 out]
                  }
                }
                n660 = for {
                  N: 32 -> [_]
                  i -> [w378]
                  n661 = for {
                    N: 5 -> [_]
                    tunnel: w378 -> [w381]
                    i -> [w380]
                    n662 = Bundle(w381, w380) -> (w382:cluster{i32, i32})  [unwired: 1 in]
                    n663 = property on="Analog_WC" class="Tbl (严格)"("Active Cell"=w382) -> (error out=w384:errorcluster)  [unwired: 2 in, 1 out]
                    n664 = property on="Analog_WC" class="Tbl (严格)"(error in=w384, "Cell BG Color"=u32 16448250) -> ()  [unwired: 1 in, 2 out]
                  }
                }
                n665 = local write "第几组数据"(w371) -> ()
                n666 = local write "第几个数据"(w371) -> ()
                n667 = local write "同步_1"(0 ("同步_2")) -> ()
                n668 = local write "数组_设定值"(w376) -> ()
                n669 = local write "bSend"(w366) -> ()
                n670 = local write "bRece"(w366) -> ()
              }
              frame #1 {
                n671 = local read "Analog_back"() -> (w392:string[][])
                n672 = local read "Analog_WC"() -> (w391:string[][])
                n673 = for {
                  tunnel: w391 -> [w428] mode=indexing
                  i -> [w427]
                  n674 = for {
                    tunnel: w428 -> [_] mode=indexing
                    tunnel: w427 -> [w432]
                    i -> [w431]
                    n675 = local read "Analog_WC"() -> (w433:string[][])
                    n676 = Replace Array Subset(array=w433, new element="", index (row)=w432, index (col)=w431) -> (w429:string[][])
                    n677 = local write "Analog_WC"(w429) -> ()
                  }
                }
                n678 = for {
                  tunnel: w392 -> [w435] mode=indexing
                  i -> [w434]
                  n679 = for {
                    tunnel: w435 -> [_] mode=indexing
                    tunnel: w434 -> [w439]
                    i -> [w438]
                    n680 = local read "Analog_back"() -> (w440:string[][])
                    n681 = Replace Array Subset(array=w440, new element="", index (row)=w439, index (col)=w438) -> (w436:string[][])
                    n682 = local write "Analog_back"(w436) -> ()
                  }
                }
                n683 = for {
                  N: 32 -> [_]
                  i -> [w394]
                  n684 = case shown="4" w394 {
                    tunnel: cluster{u32, u32}[] [{9868950, 9868950}] -> [w395 w396 w397 w398 w399 w400 w401 w402 w403 w404 w405 w406 w407 w408 w409 w410 w411 w412 w413 w414 w415 w416 w417 w418 w419 w420 w421 w422 w423 w424 w425 w426]
                    frame 0, Default {
                      n685 = property on="light_1" class="Bool (严格)"("Colors [4]"=w395) -> ()  [unwired: 2 in, 2 out]
                    }
                    frame 1 {
                      n686 = property on="light_2" class="Bool (严格)"("Colors [4]"=w396) -> ()  [unwired: 2 in, 2 out]
                    }
                    frame 2 {
                      n687 = property on="light_3" class="Bool (严格)"("Colors [4]"=w397) -> ()  [unwired: 2 in, 2 out]
                    }
                    frame 3 {
                      n688 = property on="light_4" class="Bool (严格)"("Colors [4]"=w398) -> ()  [unwired: 2 in, 2 out]
                    }
                    frame 4 {
                      n689 = property on="light_5" class="Bool (严格)"("Colors [4]"=w399) -> ()  [unwired: 2 in, 2 out]
                    }
                    frame 5 {
                      n690 = property on="light_6" class="Bool (严格)"("Colors [4]"=w400) -> ()  [unwired: 2 in, 2 out]
                    }
                    frame 6 {
                      n691 = property on="light_7" class="Bool (严格)"("Colors [4]"=w401) -> ()  [unwired: 2 in, 2 out]
                    }
                    frame 7 {
                      n692 = property on="light_8" class="Bool (严格)"("Colors [4]"=w402) -> ()  [unwired: 2 in, 2 out]
                    }
                    frame 8 {
                      n693 = property on="light_9" class="Bool (严格)"("Colors [4]"=w403) -> ()  [unwired: 2 in, 2 out]
                    }
                    frame 9 {
                      n694 = property on="light_10" class="Bool (严格)"("Colors [4]"=w404) -> ()  [unwired: 2 in, 2 out]
                    }
                    frame 10 {
                      n695 = property on="light_11" class="Bool (严格)"("Colors [4]"=w405) -> ()  [unwired: 2 in, 2 out]
                    }
                    frame 11 {
                      n696 = property on="light_12" class="Bool (严格)"("Colors [4]"=w406) -> ()  [unwired: 2 in, 2 out]
                    }
                    frame 12 {
                      n697 = property on="light_13" class="Bool (严格)"("Colors [4]"=w407) -> ()  [unwired: 2 in, 2 out]
                    }
                    frame 13 {
                      n698 = property on="light_14" class="Bool (严格)"("Colors [4]"=w408) -> ()  [unwired: 2 in, 2 out]
                    }
                    frame 14 {
                      n699 = property on="light_15" class="Bool (严格)"("Colors [4]"=w409) -> ()  [unwired: 2 in, 2 out]
                    }
                    frame 15 {
                      n700 = property on="light_16" class="Bool (严格)"("Colors [4]"=w410) -> ()  [unwired: 2 in, 2 out]
                    }
                    frame 16 {
                      n701 = property on="light_17" class="Bool (严格)"("Colors [4]"=w411) -> ()  [unwired: 2 in, 2 out]
                    }
                    frame 17 {
                      n702 = property on="light_18" class="Bool (严格)"("Colors [4]"=w412) -> ()  [unwired: 2 in, 2 out]
                    }
                    frame 18 {
                      n703 = property on="light_19" class="Bool (严格)"("Colors [4]"=w413) -> ()  [unwired: 2 in, 2 out]
                    }
                    frame 19 {
                      n704 = property on="light_20" class="Bool (严格)"("Colors [4]"=w414) -> ()  [unwired: 2 in, 2 out]
                    }
                    frame 20 {
                      n705 = property on="light_21" class="Bool (严格)"("Colors [4]"=w415) -> ()  [unwired: 2 in, 2 out]
                    }
                    frame 21 {
                      n706 = property on="light_22" class="Bool (严格)"("Colors [4]"=w416) -> ()  [unwired: 2 in, 2 out]
                    }
                    frame 22 {
                      n707 = property on="light_23" class="Bool (严格)"("Colors [4]"=w417) -> ()  [unwired: 2 in, 2 out]
                    }
                    frame 23 {
                      n708 = property on="light_24" class="Bool (严格)"("Colors [4]"=w418) -> ()  [unwired: 2 in, 2 out]
                    }
                    frame 24 {
                      n709 = property on="light_25" class="Bool (严格)"("Colors [4]"=w419) -> ()  [unwired: 2 in, 2 out]
                    }
                    frame 25 {
                      n710 = property on="light_26" class="Bool (严格)"("Colors [4]"=w420) -> ()  [unwired: 2 in, 2 out]
                    }
                    frame 26 {
                      n711 = property on="light_27" class="Bool (严格)"("Colors [4]"=w421) -> ()  [unwired: 2 in, 2 out]
                    }
                    frame 27 {
                      n712 = property on="light_28" class="Bool (严格)"("Colors [4]"=w422) -> ()  [unwired: 2 in, 2 out]
                    }
                    frame 28 {
                      n713 = property on="light_29" class="Bool (严格)"("Colors [4]"=w423) -> ()  [unwired: 2 in, 2 out]
                    }
                    frame 29 {
                      n714 = property on="light_30" class="Bool (严格)"("Colors [4]"=w424) -> ()  [unwired: 2 in, 2 out]
                    }
                    frame 30 {
                      n715 = property on="light_31" class="Bool (严格)"("Colors [4]"=w425) -> ()  [unwired: 2 in, 2 out]
                    }
                    frame 31 {
                      n716 = property on="light_32" class="Bool (严格)"("Colors [4]"=w426) -> ()  [unwired: 2 in, 2 out]
                    }
                  }
                }
              }
              frame #2 {
                n717 = for {
                  N: 32 -> [_]
                  i -> [w443]
                  n718 = disable-structure shown="禁用" {
                    frame Disabled {
                      n719 = Wait Until Next ms Multiple(millisecond multiple=u32 10 ("毫秒倍数")) -> ()  [unwired: 1 out]
                    }
                    frame Enabled {
                    }
                  }
                  n720 = for {
                    N: 6 -> [_]
                    tunnel: w443 -> [w451]
                    i -> [w448]
                    n721 = Quotient & Remainder(x=w451, y=2) -> (x-y*floor(x/y)=w449:i32)  [unwired: 1 out]
                    n722 = Equal To 0?(x=w449) -> (x = 0?=w452:bool)
                    n723 = case shown="假" w452 {
                      tunnel: [u32 16448250 u32 15723488] -> w445
                      frame False {
                      }
                      frame True {
                      }
                    }
                    n724 = Bundle(w451, w448) -> (w447:cluster{i32, i32})  [unwired: 1 in]
                    n725 = property on="Analog_WC" class="Tbl (严格)"("Active Cell"=w447) -> (error out=w446:errorcluster)  [unwired: 2 in, 1 out]
                    n726 = property on="Analog_WC" class="Tbl (严格)"(error in=w446, "Cell BG Color"=w445) -> ()  [unwired: 1 in, 2 out]
                  }
                }
              }
              frame #3 {
                n727 = local read "A_10"() -> (w483:bool)
                n728 = local read "A_11"() -> (w482:bool)
                n729 = local read "A_12"() -> (w481:bool)
                n730 = local read "A_13"() -> (w480:bool)
                n731 = local read "A_14"() -> (w479:bool)
                n732 = local read "A_15"() -> (w478:bool)
                n733 = local read "A_16"() -> (w477:bool)
                n734 = local read "A_17"() -> (w476:bool)
                n735 = local read "A_18"() -> (w475:bool)
                n736 = local read "A_19"() -> (w474:bool)
                n737 = local read "A_20"() -> (w473:bool)
                n738 = local read "A_21"() -> (w472:bool)
                n739 = local read "A_22"() -> (w471:bool)
                n740 = local read "A_23"() -> (w470:bool)
                n741 = local read "A_24"() -> (w469:bool)
                n742 = local read "A_25"() -> (w468:bool)
                n743 = local read "A_26"() -> (w467:bool)
                n744 = local read "A_27"() -> (w466:bool)
                n745 = local read "A_28"() -> (w465:bool)
                n746 = local read "A_29"() -> (w464:bool)
                n747 = local read "A_30"() -> (w463:bool)
                n748 = local read "A_31"() -> (w462:bool)
                n749 = local read "A_32"() -> (w461:bool)
                n750 = local read "A_1"() -> (w492:bool)
                n751 = local read "A_2"() -> (w491:bool)
                n752 = local read "A_3"() -> (w490:bool)
                n753 = local read "A_4"() -> (w489:bool)
                n754 = local read "A_5"() -> (w488:bool)
                n755 = local read "A_6"() -> (w487:bool)
                n756 = local read "A_7"() -> (w486:bool)
                n757 = local read "A_8"() -> (w485:bool)
                n758 = local read "A_9"() -> (w484:bool)
                n759 = Build Array(w492, w491, w490, w489, w488, w487, w486, w485, w484, w483, w482, w481, w480, w479, w478, w477, w476, w475, w474, w473, w472, w471, w470, w469, w468, w467, w466, w465, w464, w463, w462, w461) -> (w455:bool[])
                n760 = Or Array Elements(Boolean array=w455) -> (logical OR=w460:bool)
                n761 = case shown="真" w460 {
                  frame False {
                    n762 = call "显示对话框信息"() -> ()  [unwired: 10 in, 2 out]
                  }
                  frame True {
                    n763 = local write "starttest"(TRUE) -> ()
                    n764 = property on="btn_取消" class="Bool"("DisabledEnum"=T1."Disabled and Grayed Out" ("禁用")) -> ()  [unwired: 2 in, 2 out]
                  }
                }
                n765 = local write "数组_选择"(w455) -> ()
                n766 = Initialize Array(FALSE, 32 ("维数大小"), 5 ("维数大小")) -> (w456:bool[][])
                n767 = local write "合格？"(w456) -> ()
              }
            }
          }
          event "btn_全选": Value Change {
            w495 = TRUE ("单选_AD_1")
            n768 = event-data() -> ()  [unwired: 1 in, 5 out]
            n769 = local write "A_1"(w495) -> ()
            n770 = local write "A_2"(w495) -> ()
            n771 = local write "A_3"(w495) -> ()
            n772 = local write "A_4"(w495) -> ()
            n773 = local write "A_5"(w495) -> ()
            n774 = local write "A_6"(w495) -> ()
            n775 = local write "A_7"(w495) -> ()
            n776 = local write "A_8"(w495) -> ()
            n777 = local write "A_9"(w495) -> ()
            n778 = local write "A_10"(w495) -> ()
            n779 = local write "A_11"(w495) -> ()
            n780 = local write "A_12"(w495) -> ()
            n781 = local write "A_13"(w495) -> ()
            n782 = local write "A_14"(w495) -> ()
            n783 = local write "A_15"(w495) -> ()
            n784 = local write "A_16"(w495) -> ()
            n785 = local write "A_17"(w495) -> ()
            n786 = local write "A_18"(w495) -> ()
            n787 = local write "A_19"(w495) -> ()
            n788 = local write "A_20"(w495) -> ()
            n789 = local write "A_21"(w495) -> ()
            n790 = local write "A_22"(w495) -> ()
            n791 = local write "A_23"(w495) -> ()
            n792 = local write "A_24"(w495) -> ()
            n793 = local write "A_25"(w495) -> ()
            n794 = local write "A_26"(w495) -> ()
            n795 = local write "A_27"(w495) -> ()
            n796 = local write "A_28"(w495) -> ()
            n797 = local write "A_29"(w495) -> ()
            n798 = local write "A_30"(w495) -> ()
            n799 = local write "A_31"(w495) -> ()
            n800 = local write "A_32"(w495) -> ()
          }
          event "btn_反选": Value Change {
            n801 = event-data() -> ()  [unwired: 1 in, 5 out]
            n802 = local read "A_17"() -> (w527:bool)
            n803 = local read "A_18"() -> (w525:bool)
            n804 = local read "A_19"() -> (w523:bool)
            n805 = local read "A_20"() -> (w521:bool)
            n806 = local read "A_21"() -> (w519:bool)
            n807 = local read "A_22"() -> (w517:bool)
            n808 = local read "A_23"() -> (w515:bool)
            n809 = local read "A_24"() -> (w513:bool)
            n810 = local read "A_25"() -> (w511:bool)
            n811 = local read "A_26"() -> (w509:bool)
            n812 = local read "A_27"() -> (w507:bool)
            n813 = local read "A_28"() -> (w505:bool)
            n814 = local read "A_29"() -> (w503:bool)
            n815 = local read "A_30"() -> (w501:bool)
            n816 = local read "A_31"() -> (w499:bool)
            n817 = local read "A_32"() -> (w497:bool)
            n818 = local read "A_1"() -> (w559:bool)
            n819 = local read "A_2"() -> (w557:bool)
            n820 = local read "A_3"() -> (w556:bool)
            n821 = local read "A_4"() -> (w555:bool)
            n822 = local read "A_5"() -> (w554:bool)
            n823 = local read "A_6"() -> (w553:bool)
            n824 = local read "A_7"() -> (w552:bool)
            n825 = local read "A_8"() -> (w551:bool)
            n826 = local read "A_9"() -> (w550:bool)
            n827 = local read "A_10"() -> (w549:bool)
            n828 = local read "A_11"() -> (w548:bool)
            n829 = local read "A_12"() -> (w547:bool)
            n830 = local read "A_13"() -> (w546:bool)
            n831 = local read "A_14"() -> (w545:bool)
            n832 = local read "A_15"() -> (w544:bool)
            n833 = local read "A_16"() -> (w543:bool)
            n834 = Not(x=w559) -> (.not. x?=w558:bool)
            n835 = Not(x=w557) -> (.not. x?=w528:bool)
            n836 = Not(x=w556) -> (.not. x?=w529:bool)
            n837 = Not(x=w555) -> (.not. x?=w530:bool)
            n838 = Not(x=w554) -> (.not. x?=w531:bool)
            n839 = Not(x=w553) -> (.not. x?=w532:bool)
            n840 = Not(x=w552) -> (.not. x?=w533:bool)
            n841 = Not(x=w551) -> (.not. x?=w534:bool)
            n842 = Not(x=w550) -> (.not. x?=w535:bool)
            n843 = Not(x=w549) -> (.not. x?=w536:bool)
            n844 = Not(x=w548) -> (.not. x?=w537:bool)
            n845 = Not(x=w547) -> (.not. x?=w538:bool)
            n846 = Not(x=w546) -> (.not. x?=w539:bool)
            n847 = Not(x=w545) -> (.not. x?=w540:bool)
            n848 = Not(x=w544) -> (.not. x?=w541:bool)
            n849 = Not(x=w543) -> (.not. x?=w542:bool)
            n850 = Not(x=w527) -> (.not. x?=w526:bool)
            n851 = Not(x=w525) -> (.not. x?=w524:bool)
            n852 = Not(x=w523) -> (.not. x?=w522:bool)
            n853 = Not(x=w521) -> (.not. x?=w520:bool)
            n854 = Not(x=w519) -> (.not. x?=w518:bool)
            n855 = Not(x=w517) -> (.not. x?=w516:bool)
            n856 = Not(x=w515) -> (.not. x?=w514:bool)
            n857 = Not(x=w513) -> (.not. x?=w512:bool)
            n858 = Not(x=w511) -> (.not. x?=w510:bool)
            n859 = Not(x=w509) -> (.not. x?=w508:bool)
            n860 = Not(x=w507) -> (.not. x?=w506:bool)
            n861 = Not(x=w505) -> (.not. x?=w504:bool)
            n862 = Not(x=w503) -> (.not. x?=w502:bool)
            n863 = Not(x=w501) -> (.not. x?=w500:bool)
            n864 = Not(x=w499) -> (.not. x?=w498:bool)
            n865 = Not(x=w497) -> (.not. x?=w496:bool)
            n866 = local write "A_1"(w558) -> ()
            n867 = local write "A_2"(w528) -> ()
            n868 = local write "A_3"(w529) -> ()
            n869 = local write "A_4"(w530) -> ()
            n870 = local write "A_5"(w531) -> ()
            n871 = local write "A_6"(w532) -> ()
            n872 = local write "A_7"(w533) -> ()
            n873 = local write "A_8"(w534) -> ()
            n874 = local write "A_9"(w535) -> ()
            n875 = local write "A_10"(w536) -> ()
            n876 = local write "A_11"(w537) -> ()
            n877 = local write "A_12"(w538) -> ()
            n878 = local write "A_13"(w539) -> ()
            n879 = local write "A_14"(w540) -> ()
            n880 = local write "A_15"(w541) -> ()
            n881 = local write "A_16"(w542) -> ()
            n882 = local write "A_17"(w526) -> ()
            n883 = local write "A_18"(w524) -> ()
            n884 = local write "A_19"(w522) -> ()
            n885 = local write "A_20"(w520) -> ()
            n886 = local write "A_21"(w518) -> ()
            n887 = local write "A_22"(w516) -> ()
            n888 = local write "A_23"(w514) -> ()
            n889 = local write "A_24"(w512) -> ()
            n890 = local write "A_25"(w510) -> ()
            n891 = local write "A_26"(w508) -> ()
            n892 = local write "A_27"(w506) -> ()
            n893 = local write "A_28"(w504) -> ()
            n894 = local write "A_29"(w502) -> ()
            n895 = local write "A_30"(w500) -> ()
            n896 = local write "A_31"(w498) -> ()
            n897 = local write "A_32"(w496) -> ()
          }
        }
        n898 = local write "退出？"(w361) -> ()
      }
      n899 = Obtain Notifier(name (unnamed)=w168, notification data type=w168) -> (notifier out=w167:refnum<notifier>)  [unwired: 2 in, 2 out]
      n900 = while {
        tunnel: w167 -> [w280]
        stop <- w281 stop-if-true
        n901 = local read "starttest"() -> (w279:bool)
        n902 = Wait Until Next ms Multiple(millisecond multiple=u32 10 ("毫秒倍数")) -> ()  [unwired: 1 out]
        n903 = case shown="真" w279 {
          tunnel: w280 -> [_ w283]
          frame False {
          }
          frame True {
            n904 = stacked-sequence {
              tunnel: w283 -> [w285 _]
              frame #0 {
                n905 = for {
                  N: 32 -> [_]
                  tunnel: w285 -> [w287]
                  i -> [w286]
                  n906 = local read "数组_选择"() -> (w289:bool[])
                  n907 = local read "数组_设定值"() -> (w290:dbl[][])
                  n908 = local write "第几组数据"(w286) -> ()
                  n909 = Index Array(array=w289, index=w286) -> (element=w288:bool)
                  n910 = case shown="真" w288 {
                    tunnel: w286 -> [_ w297]
                    tunnel: w290 -> [_ w301]
                    tunnel: w287 -> [_ w300]
                    frame False {
                    }
                    frame True {
                      n911 = global read "试验配置信息.vi" "输出切换ID"() -> (w299:i32[])
                      n912 = global read "试验配置信息.vi" "输入切换ID"() -> (w298:i32[])
                      n913 = Index Array(array=w299, index=w297) -> (element=w294:i32)
                      n914 = Greater Or Equal To 0?(x=w294) -> (x >= 0?=w295:bool)
                      n915 = Index Array(array=w298, index=w297) -> (element=w292:i32)
                      n916 = Greater Or Equal To 0?(x=w292) -> (x >= 0?=w293:bool)
                      n917 = And(x=w295, y=w293) -> (x .and. y?=w296:bool)
                      n918 = case shown="真" w296 {
                        tunnel: w294 -> [_ w305]
                        tunnel: w292 -> [_ w304]
                        tunnel: [TRUE w303] -> w291
                        frame False {
                        }
                        frame True {
                          n919 = call "can开关切换.vi"("输入切换ID"=w304, "输出切换ID"=w305, "函数类型"=1) -> ("成功？"=w303:bool)  [unwired: 7 in]
                        }
                      }
                      n920 = case shown="真" w291 {
                        tunnel: w297 -> [_ w312]
                        tunnel: w301 -> [_ w313]
                        tunnel: w300 -> [_ w311]
                        frame False {
                          n921 = local read "第几组数据"() -> (w308:i32)
                          n922 = Increment(x=w308) -> (x+1=w307:i32)
                          n923 = Format Into String(format string="第%d路CAN切换失败！", w307) -> (resulting string=w309:string)  [unwired: 2 in, 1 out]
                          n924 = call "显示对话框信息2"("Message"=w309) -> ()  [unwired: 9 in, 2 out]
                        }
                        frame True {
                          n925 = for {
                            N: 5 -> [_]
                            tunnel: w312 -> [w318]
                            tunnel: w313 -> [w317]
                            tunnel: w311 -> [w315]
                            i -> [w316]
                            n926 = while {
                              tunnel: w318 -> [w326]
                              tunnel: w317 -> [w325]
                              tunnel: w316 -> [w324]
                              tunnel: w315 -> [w319]
                              stop <- w323 stop-if-true
                              n927 = local read "bSend"() -> (w321:bool)
                              n928 = Wait Until Next ms Multiple(millisecond multiple=u32 10 ("毫秒倍数")) -> ()  [unwired: 1 out]
                              n929 = Not(x=w321) -> (.not. x?=w320:bool)
                              n930 = case shown="真" w320 {
                                tunnel: w326 -> [_ w337]
                                tunnel: w325 -> [_ w336]
                                tunnel: w324 -> [_ w335]
                                tunnel: [w327 FALSE] -> w323
                                tunnel: w319 -> [_ w333]
                                frame False {
                                n931 = local read "bRece"() -> (w328:bool)
                                n932 = case shown="真" w328 {
                                tunnel: [FALSE w330] -> w327
                                frame False {
                                }
                                frame True {
                                n933 = stacked-sequence {
                                tunnel: [_ TRUE] -> w330
                                frame #0 {
                                w331 = FALSE
                                n934 = local write "bSend"(w331) -> ()
                                n935 = local write "bRece"(w331) -> ()
                                }
                                frame #1 {
                                }
                                }
                                }
                                }
                                }
                                frame True {
                                n936 = stacked-sequence {
                                tunnel: w337 -> [_ w346 _ _]
                                tunnel: w336 -> [_ w343 _ _]
                                tunnel: w335 -> [_ w341 _ _]
                                tunnel: w333 -> [_ _ w354 _]
                                frame #0 {
                                n937 = Wait Until Next ms Multiple(millisecond multiple=u32 200 ("毫秒倍数")) -> ()  [unwired: 1 out]
                                }
                                frame #1 {
                                # "PCI板卡下发模拟量数据"
                                n938 = global read "试验配置信息.vi" "设定输出通道"() -> (w345:u32[])
                                n939 = To Long Integer(number=w346) -> (32bit integer=w342:i32)
                                n940 = local write "第几个数据"(w341) -> ()
                                n941 = Index Array(array=w343, index (row)=w342, index (col)=w341) -> (element=w339:dbl)
                                n942 = Index Array(array=w345, index=w342) -> (element=w344:u32)
                                n943 = case shown="1" w344 {
                                tunnel: [w350 w353] -> w340
                                tunnel: w339 -> [w348 w351]
                                frame 0, Default {
                                n944 = Build Array(w348, 0.0) -> (w350:dbl[])
                                }
                                frame 1 {
                                n945 = Build Array(0.0, w351) -> (w353:dbl[])
                                }
                                }
                                n946 = call "Convert to Dynamic Data"("Array"=w340) -> ("Dynamic Data Type"=w347:dynamicdata)  [unwired: 3 out]
                                n947 = call "DAQNavi Assistant"("data in(DDT)"=w347) -> ()  [unwired: 2 in, 17 out]
                                }
                                frame #2 {
                                n948 = local write "同步_1"(1 ("y")) -> ()
                                n949 = Send Notification(notification="NumCheck" ("通知"), notifier=w354) -> ()  [unwired: 1 in, 2 out]
                                }
                                frame #3 {
                                n950 = local write "bSend"(TRUE) -> ()
                                }
                                }
                                }
                              }
                            }
                          }
                        }
                      }
                    }
                  }
                }
              }
              frame #1 {
                n951 = local write "starttest"(FALSE) -> ()
                n952 = property on="btn_取消" class="Bool"("DisabledEnum"=T1."Enabled" ("禁用")) -> ()  [unwired: 2 in, 2 out]
              }
            }
          }
        }
        n953 = local read "退出？"() -> (w281:bool)
      }
      n954 = Obtain Notifier(name (unnamed)=w165, notification data type=w165) -> (notifier out=w164:refnum<notifier>)  [unwired: 2 in, 2 out]
      n955 = while {
        tunnel: w164 -> [w172]
        tunnel: [w171] -> w166
        stop <- w175 stop-if-true
        n956 = Wait Until Next ms Multiple(millisecond multiple=u32 10 ("毫秒倍数")) -> ()  [unwired: 1 out]
        n957 = Wait on Notification(notifier=w172, timeout in ms (-1)=10 ("超时毫秒(-1)")) -> (notifier out=w171:refnum<notifier>, notification=w170:string)  [unwired: 2 in, 2 out]
        n958 = Equal?(x=w170, y="NumCheck" ("通知")) -> (x = y?=w173:bool)
        n959 = case shown="真" w173 {
          frame False {
          }
          frame True {
            n960 = call "DAQNavi Assistant2"() -> ("error out"=w180:errorcluster, "data out(DDT)"=w181:dynamicdata)  [unwired: 2 in, 16 out]
            n961 = Unbundle By Name(w180) -> ("status"=w178:bool)
            n962 = case shown="真" w178 {
              frame False {
              }
              frame True {
                n963 = call "超时"() -> ()  [unwired: 10 in, 2 out]
                n964 = local write "同步_1"(0 ("同步_1")) -> ()
              }
            }
            n965 = call "从动态数据转换"("Dynamic Data Type"=w181) -> ("Array"=w182:dbl[])  [unwired: 3 in]
            n966 = To Single Precision Float(number=w182) -> (single precision float=w177:sgl[])
            n967 = Not(x=w178) -> (.not. x?=w179:bool)
            n968 = case shown="真" w179 {
              tunnel: w177 -> [_ w184]
              frame False {
              }
              frame True {
                n969 = stacked-sequence {
                  tunnel: w184 -> [w211 _ _ _]
                  frame #0 {
                    n970 = global read "试验配置信息.vi" "设定输入通道"() -> (w210:u32[])
                    n971 = local read "第几组数据"() -> (w209:i32)
                    n972 = local read "第几组数据"() -> (w197:i32)
                    n973 = global read "试验配置信息.vi" "允许误差"() -> (w198:dbl[])
                    n974 = global read "试验配置信息.vi" "参数A1"() -> (w205:dbl[])
                    n975 = global read "试验配置信息.vi" "参数A2"() -> (w204:dbl[])
                    n976 = global read "试验配置信息.vi" "Max"() -> (w199:dbl[])
                    n977 = global read "试验配置信息.vi" "min"() -> (w200:dbl[])
                    n978 = local read "第几个数据"() -> (w207:i32)
                    n979 = local read "数组_设定值"() -> (w221:dbl[][])
                    n980 = Index Array(array=w210, index=w209) -> (element=w208:u32)
                    n981 = Index Array(array=w211, index=w208) -> (element=w189:sgl)
                    n982 = Index Array(array=w199, index=w197) -> (element=w196:dbl)
                    n983 = Index Array(array=w200, index=w197) -> (element=w195:dbl)
                    n984 = Index Array(array=w205, index=w197) -> (element=w187:dbl)
                    n985 = Index Array(array=w204, index=w197) -> (element=w203:dbl)
                    n986 = Index Array(array=w198, index=w197) -> (element=w193:dbl)
                    n987 = Subtract(x=w196, y=w195) -> (x-y=w194:dbl)
                    n988 = local read "Analog_back"() -> (w215:string[][])
                    n989 = local read "第几个数据"() -> (w212:i32)
                    n990 = Absolute Value(x=w194) -> (abs(x)=w186:dbl)
                    n991 = Index Array(array=w221, index (row)=w197, index (col)=w207) -> (element=w206:dbl)
                    n992 = local read "数组_选择"() -> (w202:bool[])
                    n993 = Number To Fractional String(number=w189, precision (6)=i16 3 ("精度(6)")) -> (F-format string=w188:string)  [unwired: 2 in]
                    n994 = call "函数公式.vi"("参数 b"=w203, "参数 a"=w187, "设定值 1"=w206) -> ("y"=w201:dbl)  [unwired: 5 in, 1 out]
                    n995 = Multiply(x=w187, y=w186) -> (x*y=w185:dbl)
                    n996 = Replace Array Subset(array=w215, new element=w188, index (row)=w209, index (col)=w212) -> (w214:string[][])
                    n997 = call "误差计算.vi"("选择?"=w202, "允许误差"=w193, "模拟量量程范围"=w185, "设定值_1"=w201, "反馈值_1"=w189) -> ("字符串_误差_1"=w191:string, "合格_1?"=w192:bool)  [unwired: 4 in, 1 out]
                    n998 = local write "Analog_back"(w214) -> ()
                    n999 = local read "第几个数据"() -> (w213:i32)
                    n1000 = local read "Analog_WC"() -> (w220:string[][])
                    n1001 = local read "第几组数据"() -> (w218:i32)
                    n1002 = Replace Array Subset(array=w220, new element=w191, index (row)=w218, index (col)=w213) -> (w219:string[][])
                    n1003 = local read "合格？"() -> (w216:bool[][])
                    n1004 = local write "Analog_WC"(w219) -> ()
                    n1005 = Replace Array Subset(array=w216, new element=w192, index (row)=w218, index (col)=w213) -> (w217:bool[][])
                    n1006 = local write "合格？"(w217) -> ()
                  }
                  frame #1 {
                    n1007 = local read "合格？"() -> (w226:bool[][])
                    n1008 = local read "第几组数据"() -> (w223:i32)
                    n1009 = Index Array(array=w226, index (row)=w223) -> (element=w228:bool[])  [unwired: 1 in]
                    n1010 = And Array Elements(Boolean array=w228) -> (logical AND=w225:bool)
                    n1011 = local read "数组_选择"() -> (w224:bool[])
                    n1012 = Index Array(array=w224, index=w223) -> (element=w222:bool)
                    n1013 = case shown="真" w222 {
                      tunnel: [cluster{u32, u32}[] [{12369084, 12369084}] w231] -> w227
                      tunnel: w225 -> [_ w230]
                      frame False {
                      }
                      frame True {
                        n1014 = case shown="真" w230 {
                          tunnel: [cluster{u32, u32}[] [{16730410, 16711680}] cluster{u32, u32}[] [{61205, 6618880}]] -> w231
                          frame False {
                          }
                          frame True {
                          }
                        }
                      }
                    }
                    n1015 = case shown="31" w223 {
                      tunnel: w227 -> [w234 w235 w236 w237 w238 w239 w240 w241 w242 w243 w244 w245 w246 w247 w248 w249 w250 w251 w252 w253 w254 w255 w256 w257 w258 w259 w260 w261 w262 w263 w264 w265]
                      frame 0, Default {
                        n1016 = property on="light_1" class="Bool (严格)"("Colors [4]"=w234) -> ()  [unwired: 2 in, 2 out]
                      }
                      frame 1 {
                        n1017 = property on="light_2" class="Bool (严格)"("Colors [4]"=w235) -> ()  [unwired: 2 in, 2 out]
                      }
                      frame 2 {
                        n1018 = property on="light_3" class="Bool (严格)"("Colors [4]"=w236) -> ()  [unwired: 2 in, 2 out]
                      }
                      frame 3 {
                        n1019 = property on="light_4" class="Bool (严格)"("Colors [4]"=w237) -> ()  [unwired: 2 in, 2 out]
                      }
                      frame 4 {
                        n1020 = property on="light_5" class="Bool (严格)"("Colors [4]"=w238) -> ()  [unwired: 2 in, 2 out]
                      }
                      frame 5 {
                        n1021 = property on="light_6" class="Bool (严格)"("Colors [4]"=w239) -> ()  [unwired: 2 in, 2 out]
                      }
                      frame 6 {
                        n1022 = property on="light_7" class="Bool (严格)"("Colors [4]"=w240) -> ()  [unwired: 2 in, 2 out]
                      }
                      frame 7 {
                        n1023 = property on="light_8" class="Bool (严格)"("Colors [4]"=w241) -> ()  [unwired: 2 in, 2 out]
                      }
                      frame 8 {
                        n1024 = property on="light_9" class="Bool (严格)"("Colors [4]"=w242) -> ()  [unwired: 2 in, 2 out]
                      }
                      frame 9 {
                        n1025 = property on="light_10" class="Bool (严格)"("Colors [4]"=w243) -> ()  [unwired: 2 in, 2 out]
                      }
                      frame 10 {
                        n1026 = property on="light_11" class="Bool (严格)"("Colors [4]"=w244) -> ()  [unwired: 2 in, 2 out]
                      }
                      frame 11 {
                        n1027 = property on="light_12" class="Bool (严格)"("Colors [4]"=w245) -> ()  [unwired: 2 in, 2 out]
                      }
                      frame 12 {
                        n1028 = property on="light_13" class="Bool (严格)"("Colors [4]"=w246) -> ()  [unwired: 2 in, 2 out]
                      }
                      frame 13 {
                        n1029 = property on="light_14" class="Bool (严格)"("Colors [4]"=w247) -> ()  [unwired: 2 in, 2 out]
                      }
                      frame 14 {
                        n1030 = property on="light_15" class="Bool (严格)"("Colors [4]"=w248) -> ()  [unwired: 2 in, 2 out]
                      }
                      frame 15 {
                        n1031 = property on="light_16" class="Bool (严格)"("Colors [4]"=w249) -> ()  [unwired: 2 in, 2 out]
                      }
                      frame 16 {
                        n1032 = property on="light_17" class="Bool (严格)"("Colors [4]"=w250) -> ()  [unwired: 2 in, 2 out]
                      }
                      frame 17 {
                        n1033 = property on="light_18" class="Bool (严格)"("Colors [4]"=w251) -> ()  [unwired: 2 in, 2 out]
                      }
                      frame 18 {
                        n1034 = property on="light_19" class="Bool (严格)"("Colors [4]"=w252) -> ()  [unwired: 2 in, 2 out]
                      }
                      frame 19 {
                        n1035 = property on="light_20" class="Bool (严格)"("Colors [4]"=w253) -> ()  [unwired: 2 in, 2 out]
                      }
                      frame 20 {
                        n1036 = property on="light_21" class="Bool (严格)"("Colors [4]"=w254) -> ()  [unwired: 2 in, 2 out]
                      }
                      frame 21 {
                        n1037 = property on="light_22" class="Bool (严格)"("Colors [4]"=w255) -> ()  [unwired: 2 in, 2 out]
                      }
                      frame 22 {
                        n1038 = property on="light_23" class="Bool (严格)"("Colors [4]"=w256) -> ()  [unwired: 2 in, 2 out]
                      }
                      frame 23 {
                        n1039 = property on="light_24" class="Bool (严格)"("Colors [4]"=w257) -> ()  [unwired: 2 in, 2 out]
                      }
                      frame 24 {
                        n1040 = property on="light_25" class="Bool (严格)"("Colors [4]"=w258) -> ()  [unwired: 2 in, 2 out]
                      }
                      frame 25 {
                        n1041 = property on="light_26" class="Bool (严格)"("Colors [4]"=w259) -> ()  [unwired: 2 in, 2 out]
                      }
                      frame 26 {
                        n1042 = property on="light_27" class="Bool (严格)"("Colors [4]"=w260) -> ()  [unwired: 2 in, 2 out]
                      }
                      frame 27 {
                        n1043 = property on="light_28" class="Bool (严格)"("Colors [4]"=w261) -> ()  [unwired: 2 in, 2 out]
                      }
                      frame 28 {
                        n1044 = property on="light_29" class="Bool (严格)"("Colors [4]"=w262) -> ()  [unwired: 2 in, 2 out]
                      }
                      frame 29 {
                        n1045 = property on="light_30" class="Bool (严格)"("Colors [4]"=w263) -> ()  [unwired: 2 in, 2 out]
                      }
                      frame 30 {
                        n1046 = property on="light_31" class="Bool (严格)"("Colors [4]"=w264) -> ()  [unwired: 2 in, 2 out]
                      }
                      frame 31 {
                        n1047 = property on="light_32" class="Bool (严格)"("Colors [4]"=w265) -> ()  [unwired: 2 in, 2 out]
                      }
                    }
                  }
                  frame #2 {
                    (unwired) 32
                    n1048 = local read "第几组数据"() -> (w267:i32)
                    n1049 = local read "第几个数据"() -> (w270:i32)
                    n1050 = local read "合格？"() -> (w271:bool[][])
                    n1051 = local read "数组_选择"() -> (w269:bool[])
                    n1052 = Index Array(array=w271, index (row) #1=w267, index (col) #1=w270, index (col) #2=w270) -> (element #1=w268:bool)  [unwired: 1 in, 1 out]
                    n1053 = Index Array(array=w269, index=w267) -> (element=w266:bool)
                    n1054 = case shown="真" w266 {
                      tunnel: w270 -> [_ w275]
                      tunnel: w268 -> [_ w274]
                      tunnel: w267 -> [_ w273]
                      frame False {
                      }
                      frame True {
                        n1055 = call "误差表格颜色.vi"("合格？"=w274, "第几组"=w273) -> ("颜色"=w272:u32)  [unwired: 9 in]
                        n1056 = Bundle("第几组数据"=w273, "第几个数据"=w275) -> (w277:cluster{"第几组数据":i32, "第几个数据":i32})  [unwired: 1 in]
                        n1057 = property on="Analog_WC" class="Tbl (严格)"("Active Cell"=w277) -> (error out=w276:errorcluster)  [unwired: 2 in, 1 out]
                        n1058 = property on="Analog_WC" class="Tbl (严格)"(error in=w276, "Cell BG Color"=w272) -> ()  [unwired: 1 in, 2 out]
                      }
                    }
                  }
                  frame #3 {
                    n1059 = local write "bRece"(TRUE) -> ()
                  }
                }
              }
            }
          }
        }
        n1060 = local read "退出？"() -> (w175:bool)
      }
      n1061 = Release Notifier(notifier=w166) -> ()  [unwired: 2 in, 3 out]
    }
  }
  n1062 = disable-structure shown="禁用" {
    frame Disabled {
      n1063 = for {
        N: 32 -> [_]
        i -> [w562]
        n1064 = for {
          N: 6 -> [_]
          tunnel: w562 -> [w569]
          i -> [w566]
          n1065 = Quotient & Remainder(x=w569, y=2) -> (x-y*floor(x/y)=w567:i32)  [unwired: 1 out]
          n1066 = Equal To 0?(x=w567) -> (x = 0?=w570:bool)
          n1067 = case shown="假" w570 {
            tunnel: [u32 16448250 u32 15723488] -> w563
            frame False {
            }
            frame True {
            }
          }
          n1068 = Bundle(w569, w566) -> (w565:cluster{i32, i32})  [unwired: 1 in]
          n1069 = property on="Analog_WC" class="Tbl (严格)"("Active Cell"=w565) -> (error out=w564:errorcluster)  [unwired: 2 in, 1 out]
          n1070 = property on="Analog_WC" class="Tbl (严格)"(error in=w564, "Cell BG Color"=w563) -> ()  [unwired: 1 in, 2 out]
        }
      }
    }
    frame Enabled {
    }
  }
  n1071 = disable-structure shown="禁用" {
    frame Disabled {
      n1072 = Initialize Array("测试", 32 ("维数大小")) -> (w574:string[])
      n1073 = global write "试验配置信息.vi" "名称"(w574) -> ()
    }
    frame Enabled {
    }
  }
